vi "main.vi"() -> ()   [LabVIEW 2022 SP3]
uses:
  drawPlate.lvlib
  subvis.lvlib
panel:
  out "x > 0?":bool
  out "depth_max":i32
  out "PowerOff":bool
  in  "GameOver":bool caption="OK"
  out "returnValue":dbl
  out "MoveY":i32
  out "MoveX":i32
  out "nMoves":i32
  in  "pressedJ":i32=21414112
  in  "pressedI":i32=21414112
  out "result":i32
  in  "currentState.pos":i32[][](array[numeric])
  in  "currentState.exist":i32[][](array[numeric])
  in  "availables":i32[][](array[numeric])
  in  "Turn":i32
  in  "mode/difficulty":i32
  out "Tab Control":enum32{"menu", "board"}(tab)
  in  "OL(continue)":bool
  in  "OL(client,white)":bool
  in  "EVE":bool
  in  "OL(host,black)":bool
  in  "PVE":bool
  in  "PVP":bool
  out "mode":string
  in  "7 1":bool
  in  "7 0":bool
  in  "6 1":bool
  in  "6 0":bool
  in  "5 1":bool
  in  "5 0":bool
  in  "4 1":bool
  in  "4 0":bool
  in  "3 1":bool
  in  "3 0":bool
  in  "2 1":bool
  in  "2 0":bool
  in  "1 1":bool
  in  "1 0":bool
  in  "0 1":bool
  in  "7 7":bool
  in  "7 6":bool
  in  "7 5":bool
  in  "7 4":bool
  in  "7 3":bool
  in  "7 2":bool
  in  "6 7":bool
  in  "6 6":bool
  in  "6 5":bool
  in  "6 4":bool
  in  "6 3":bool
  in  "6 2":bool
  in  "5 7":bool
  in  "5 6":bool
  in  "5 5":bool
  in  "5 4":bool
  in  "5 3":bool
  in  "5 2":bool
  in  "4 7":bool
  in  "4 6":bool
  in  "4 5":bool
  in  "4 4":bool
  in  "4 3":bool
  in  "4 2":bool
  in  "3 7":bool
  in  "3 6":bool
  in  "3 5":bool
  in  "3 4":bool
  in  "3 3":bool
  in  "3 2":bool
  in  "2 7":bool
  in  "2 6":bool
  in  "2 5":bool
  in  "2 4":bool
  in  "2 3":bool
  in  "2 2":bool
  in  "0 7":bool
  in  "0 6":bool
  in  "0 5":bool
  in  "0 4":bool
  in  "0 3":bool
  in  "0 2":bool
  in  "1 7":bool
  in  "1 6":bool
  in  "1 5":bool
  in  "1 4":bool
  in  "1 3":bool
  in  "1 2":bool
  in  "0 0":bool
  out "board":picture
  out "Who's turn":string
  in  "GiveUp?":bool
  out "getFromNet":bool
  out "putToNet":bool
  # "等待對方中"
  # "資料上傳中"
  # "連線模式:此二任一亮著代\n表正在將資料上傳或是等\n待下載資料，請勿急著下\n下一手，會當掉。"
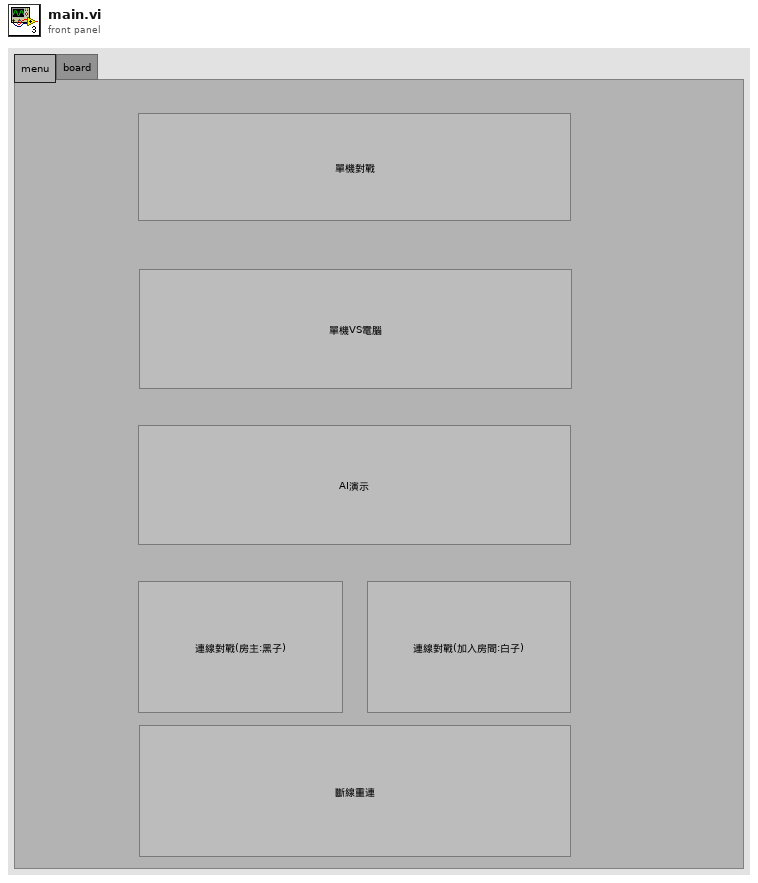
[diagram p1: front panel]
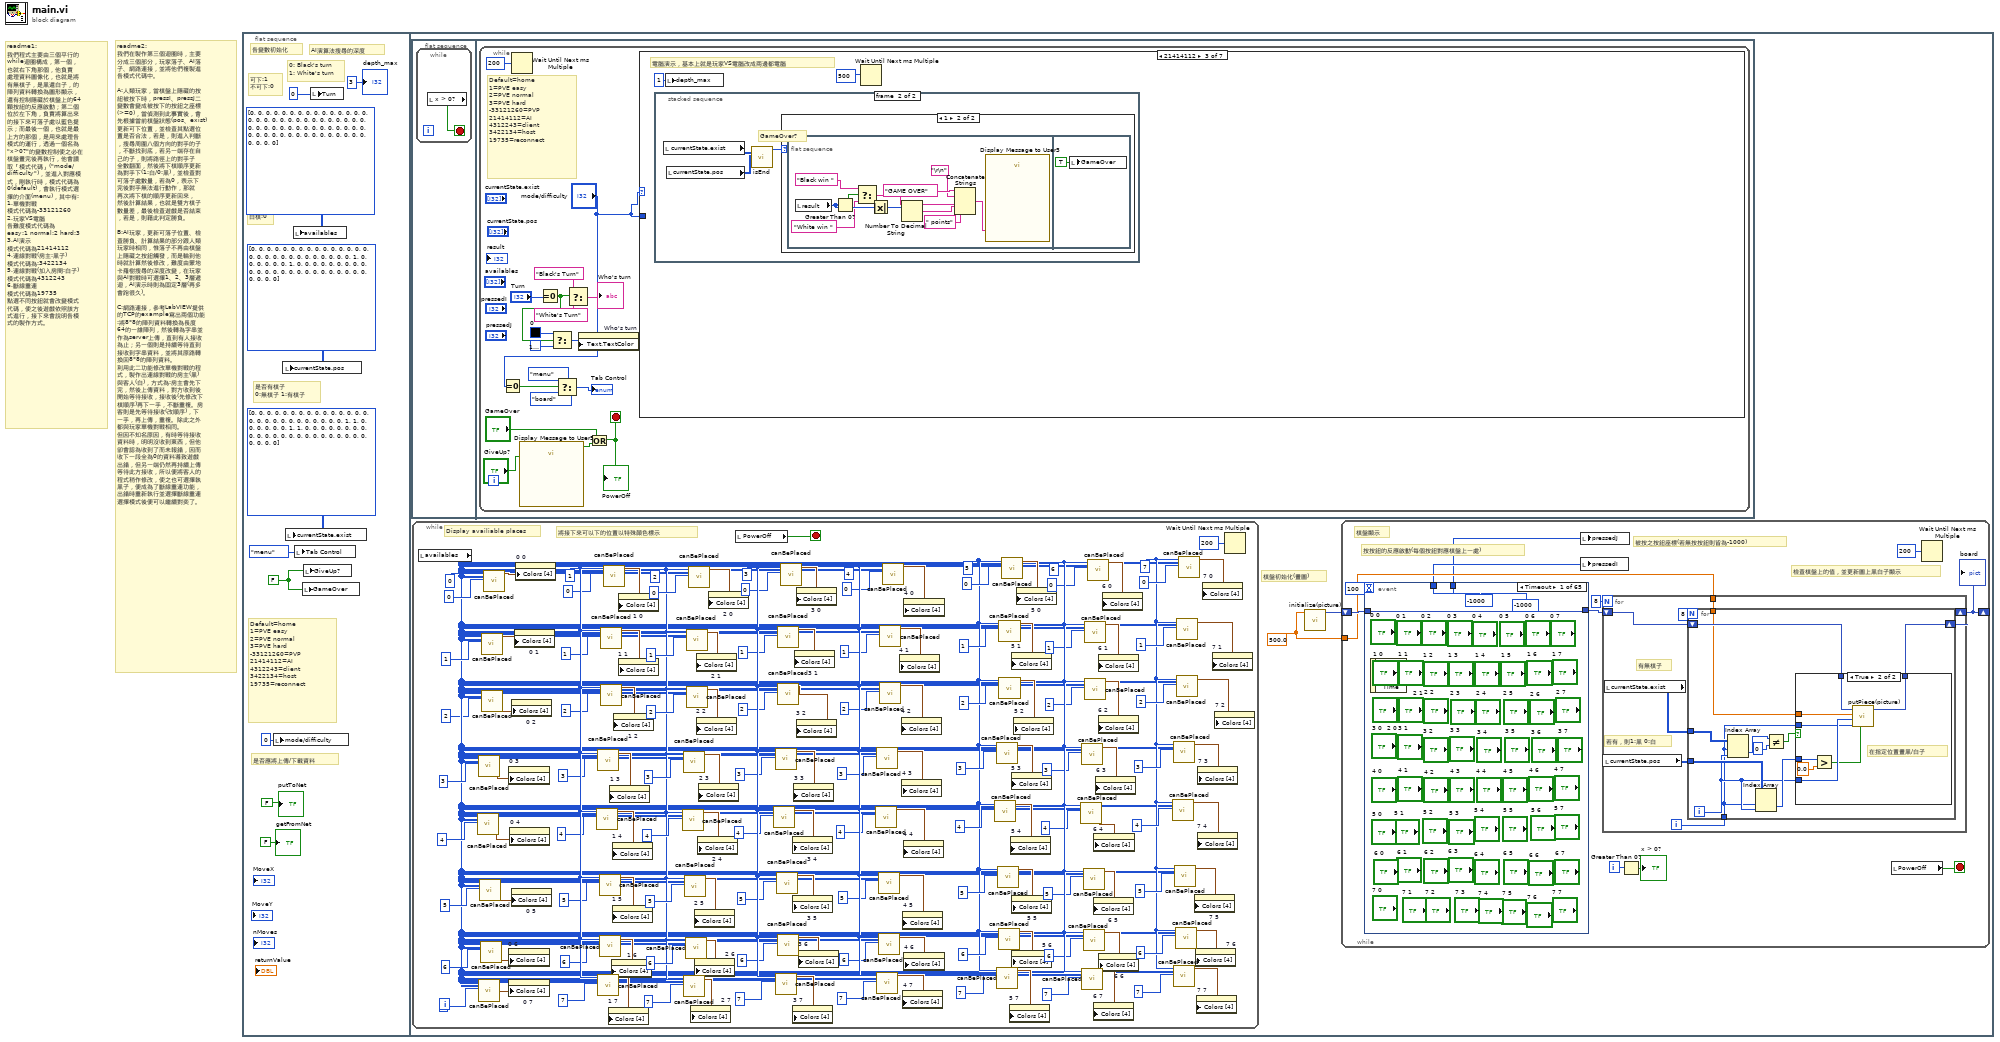
[diagram p0: block diagram]
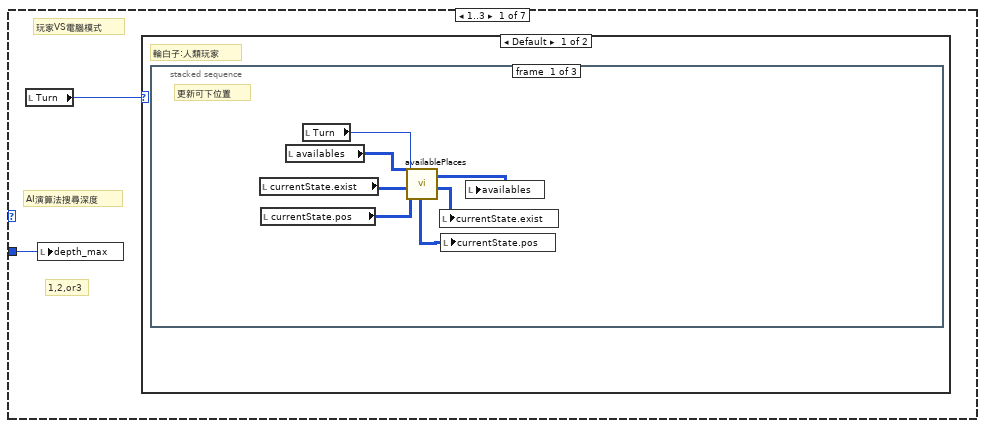
[diagram p2: hidden frame]
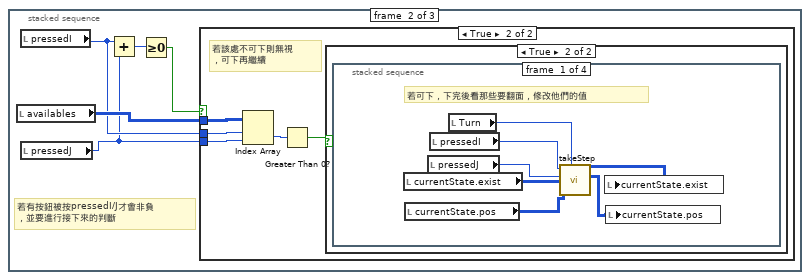
[diagram p3: hidden frame]
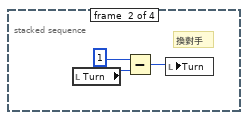
[diagram p6: hidden frame]
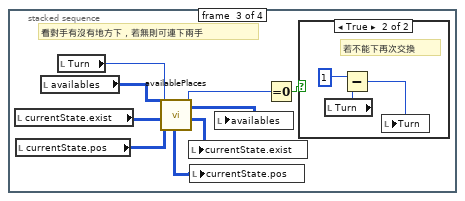
[diagram p7: hidden frame]
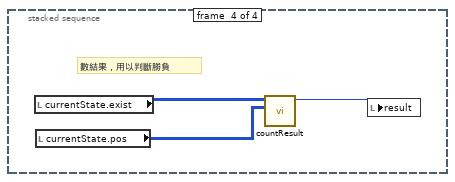
[diagram p9: hidden frame]
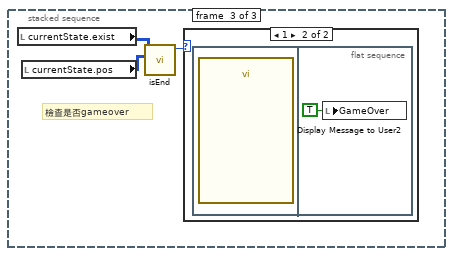
[diagram p10: hidden frame]
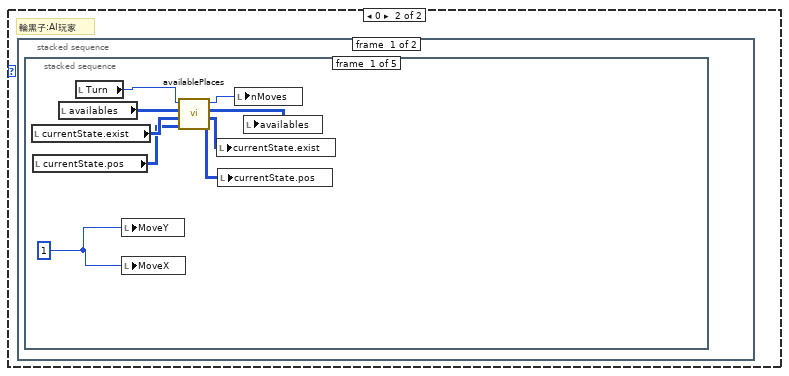
[diagram p12: hidden frame]
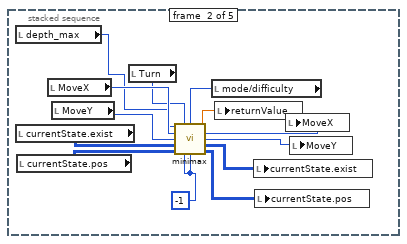
[diagram p13: hidden frame]
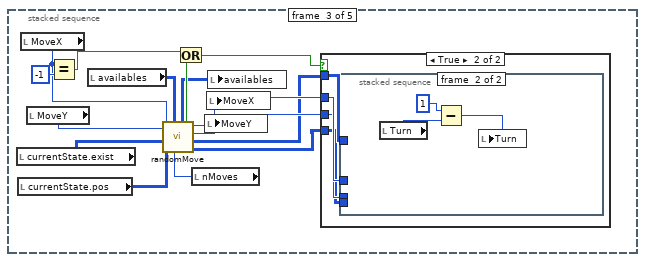
[diagram p14: hidden frame]
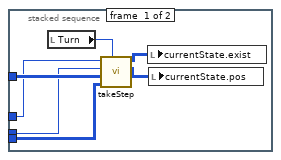
[diagram p16: hidden frame]
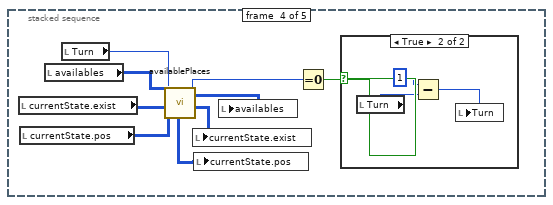
[diagram p17: hidden frame]
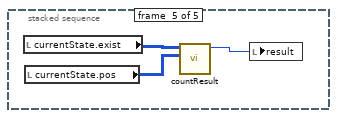
[diagram p19: hidden frame]
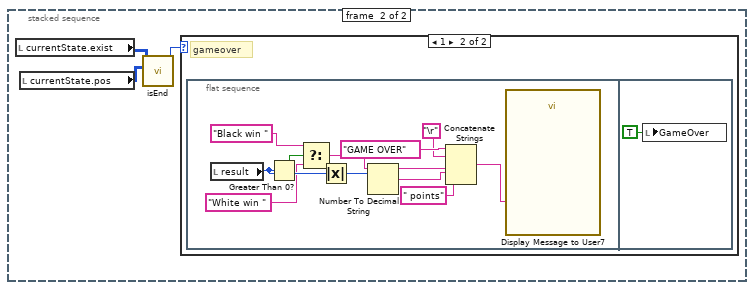
[diagram p20: hidden frame]
diagram:
  # "readme2:\n我們在製作第三個迴圈時，主要\n分成三個部分，玩家落子、AI落\n子、網路連接，並將他們複製進\n各模式代碼中。\n\nA:人類玩家，當棋盤上隱藏的按\n紐被按下時，pressI、pressJ二\n變數會變成被按下的按鈕之座標\n(>=0)，當偵測到此事實後，會\n先根據當前棋盤狀態(pos、exist)\n更新可下位置，並檢查其點選位\n置是否合法，若是，則進入判斷\n，搜尋周圍八個方向的對手的子\n，不斷找到底，若另一端存在自\n己的子，則將路徑上的對手子\n全數翻面，然後將下棋順序更新\n為對手下(1:白/0:黑)，並檢查對\n可落子處數量，若為0，表示下\n完後對手無法進行動作，那就\n再次將下棋的順序更新回來，\n然後計算結果，也就是雙方棋子\n數量差，最後檢查遊戲是否結束\n，若是，則藉此判定勝負。\n\nB:AI玩家，更新可落子位置、檢\n查勝負、計算結果的部分跟人類\n玩家時相同，惟落子不再由棋盤\n上隱藏之按鈕觸發，而是輪到他\n時就計算然後修改，難度由蒙地\n卡羅樹搜尋的深度改變，在玩家\n與AI對戰時可選擇1、2、3層遞\n迴，AI演示時則為固定3層(再多\n會跑很久)。\n\nC:網路連接，參考LabVIEW提供\n的TCP的example寫出兩個功能\n:將8*8的陣列資料轉換為長度\n64的一維陣列，然後轉為字串並\n作為server上傳，直到有人接收\n為止；另一個則是持續等待直到\n接收到字串資料，並將其原路轉\n換回8*8的陣列資料。\n利用此二功能修改單機對戰的程\n式，製作出連線對戰的房主(黑)\n與客人(白)，方式為:房主會先下\n完，然後上傳資料，對方收到後\n開始等待接收，接收後(先修改下\n棋順序)再下一手，不斷重複。房\n客則是先等待接收(改順序)，下\n一手，再上傳，重複。除此之外\n都與玩家單機對戰相同。\n但因不知名原因，有時等待接收\n資料時，明明沒收到東西，但他\n卻會認為收到了而未報錯，因而\n收下一段全為0的資料導致遊戲\n出錯，但另一端仍然再持續上傳\n等待此方接收，所以便將客人的\n程式稍作修改，使之也可選擇執\n黑子，便成為了斷線重連功能，\n出錯時重新執行並選擇斷線重連\n選擇模式後便可以繼續對奕了。"
  # "readme1:\n我們程式主要由三個平行的\nwhile迴圈構成，第一個，\n也就右下角那個，他負責\n處理資料圖像化，也就是將\n有無棋子，是黑還白子，的\n陣列資料轉換為圖形顯示，\n還有控制隱藏於棋盤上的64\n顆按紐的反應啟動；第二個\n位於左下角，負責將算出來\n的接下來可落子處以藍色提\n示；而最後一個，也就是最\n上方的那個，是用來處理各\n模式的運行，透過一個名為\n\"x>0?\"的變數控制使之必在\n棋盤畫完後再執行，他會讀\n取「模式代碼」(\"mode/\ndifficulty\")，並進入對應模\n式，剛執行時，模式代碼為\n0(default)，會執行模式選\n擇的介面(menu)，其中有:\n1.單機對戰\n模式代碼為-33121260\n2.玩家VS電腦\n各難度模式代碼為\neasy:1 normal:2 hard:3\n3.AI演示\n模式代碼為21414112\n4.連線對戰(房主:黑子)\n模式代碼為:3422134\n5.連線對戰(加入房間:白子)\n模式代碼為4312243\n6.斷線重連\n模式代碼為19735\n點選不同按鈕就會改變模式\n代碼，使之後遊戲依照該方\n式進行，接下來會說明各模\n式的製作方式。"
  n1 = flat-sequence {
    frame #0 {
      w7 = FALSE ("powerOff")
      # "是否應將上傳/下載資料"
      # "可下:1\n不可下:0"
      # "Default=home\n1=PVE easy\n2=PVE normal\n3=PVE hard\n-33121260=PVP\n21414112=AI\n4312243=client\n3422134=host\n19735=reconnect"
      # "各變數初始化"
      # "AI演算法搜尋的深度"
      # "0: Black's turn\n1: White's turn"
      # "黑棋:1\n白棋:0"
      # "是否有棋子\n0:無棋子 1:有棋子"
      n2 = local write "mode/difficulty"(0 ("mode/difficulty")) -> ()
      n3 = local write "currentState.pos"(i32[][] [[0, 0, 0, 0, 0, 0, 0, 0], [0, 0, 0, 0, 0, 0, 0, 0], [0, 0, 0, 0, 0, 0, 0, 0], [0, 0, 0, 0, 1, 0, 0, 0], [0, 0, 0, 1, 0, 0, 0, 0], [0, 0, 0, 0, 0, 0, 0, 0], [0, 0, 0, 0, 0, 0, 0, 0], [0, 0, 0, 0, 0, 0, 0, 0]] ("value")) -> ()
      n4 = local write "currentState.exist"(i32[][] [[0, 0, 0, 0, 0, 0, 0, 0], [0, 0, 0, 0, 0, 0, 0, 0], [0, 0, 0, 0, 0, 0, 0, 0], [0, 0, 0, 1, 1, 0, 0, 0], [0, 0, 0, 1, 1, 0, 0, 0], [0, 0, 0, 0, 0, 0, 0, 0], [0, 0, 0, 0, 0, 0, 0, 0], [0, 0, 0, 0, 0, 0, 0, 0]] ("value")) -> ()
      n5 = local write "availables"(i32[][] [[0, 0, 0, 0, 0, 0, 0, 0], [0, 0, 0, 0, 0, 0, 0, 0], [0, 0, 0, 0, 0, 0, 0, 0], [0, 0, 0, 0, 0, 0, 0, 0], [0, 0, 0, 0, 0, 0, 0, 0], [0, 0, 0, 0, 0, 0, 0, 0], [0, 0, 0, 0, 0, 0, 0, 0], [0, 0, 0, 0, 0, 0, 0, 0]] ("value")) -> ()
      n6 = local write "Tab Control"(enum32{"menu", "board"}."menu" ("Tab Control")) -> ()
      n7 = local write "GameOver"(w7) -> ()
      n8 = local write "GiveUp?"(w7) -> ()
      n9 = local write "Turn"(0 ("redTurn")) -> ()
      "depth_max" <- 3 ("depth_max")
      "getFromNet" <- FALSE ("getFromNet")
      "putToNet" <- FALSE ("putToNet")
    }
    frame #1 {
      w11 = 500.0 ("picture size")
      # "棋盤初始化(畫圖)"
      n10 = flat-sequence {
        frame #0 {
          n11 = while {
            stop <- w152 stop-if-true
            n12 = local read "x > 0?"() -> (w152:bool)
          }
        }
        frame #1 {
          n13 = while {
            stop <- w163 stop-if-true
            # "Default=home\n1=PVE easy\n2=PVE normal\n3=PVE hard\n-33121260=PVP\n21414112=AI\n4312243=client\n3422134=host\n19735=reconnect"
            n14 = Equal To 0?(x="mode/difficulty") -> (x = 0?=w168:bool)
            n15 = Wait Until Next ms Multiple(millisecond multiple=u32 200) -> ()  [unwired: 1 out]
            n16 = call "Display Message to User5"("Enable"="GiveUp?") -> ("OK"=w165:bool)  [unwired: 9 in, 1 out]
            n17 = Equal To 0?(x="Turn") -> (x = 0?=w158:bool)
            n18 = Select(t=u32 0 ("Text.Text Colors:Text Color"), s=w158, f=u32 16777225 ("Text.Text Colors:Text Color")) -> (s? t:f=w157:u32)
            n19 = Select(t=enum32{"menu", "board"}."menu" ("Tab Control"), s=w168, f=enum32{"menu", "board"}."board" ("Tab Control")) -> (s? t:f=→"Tab Control":enum32{"menu", "board"})
            n20 = Select(t="Black's Turn", s=w158, f="White's Turn") -> (s? t:f=→"Who's turn":string)
            n21 = property on="Who's turn" class="Str"("Text.TextColor"=w157) -> ()  [unwired: 2 in, 2 out]
            n22 = Or(x="GameOver", y=w165) -> (x .or. y?=w163:bool)
            "PowerOff" <- w163
            n23 = case shown="21414112" "mode/difficulty" {
              tunnel: "mode/difficulty" -> [w171 _ _ _ _ _ _]
              frame 1..3 {
                # "1,2,or3"
                # "AI演算法搜尋深度"
                # "玩家VS電腦模式"
                n24 = local read "Turn"() -> (w172:i32)
                n25 = local write "depth_max"(w171) -> ()
                n26 = case shown="Default" w172 {
                  frame Default {
                    # "輪白子:人類玩家"
                    n27 = stacked-sequence {
                      frame #0 {
                        # "更新可下位置"
                        n28 = local read "currentState.exist"() -> (w174:i32[][])
                        n29 = local read "currentState.pos"() -> (w173:i32[][])
                        n30 = local read "availables"() -> (w175:i32[][])
                        n31 = local read "Turn"() -> (w176:i32)
                        n32 = call "availablePlaces.vi"("pos"=w173, "exist"=w174, "available"=w175, "redTurn"=w176) -> ("posNew"=w179:i32[][], "existNew"=w178:i32[][], "availableNew"=w177:i32[][])  [unwired: 4 in, 1 out]
                        n33 = local write "currentState.exist"(w178) -> ()
                        n34 = local write "currentState.pos"(w179) -> ()
                        n35 = local write "availables"(w177) -> ()
                      }
                      frame #1 {
                        # "若有按鈕被按pressedI/J才會非負\n，並要進行接下來的判斷"
                        n36 = local read "availables"() -> (w183:i32[][])
                        n37 = local read "pressedI"() -> (w181:i32)
                        n38 = local read "pressedJ"() -> (w180:i32)
                        n39 = Add(x=w181, y=w180) -> (x+y=w184:i32)
                        n40 = Greater Or Equal To 0?(x=w184) -> (x >= 0?=w182:bool)
                        n41 = case shown="True" w182 {
                          tunnel: w183 -> [_ w189]
                          tunnel: w181 -> [_ w188]
                          tunnel: w180 -> [_ w187]
                          frame False {
                          }
                          frame True {
                            # "若該處不可下則無視\n，可下再繼續"
                            n42 = Index Array(array=w189, index (row)=w188, index (col)=w187) -> (element=w185:i32)
                            n43 = Greater Than 0?(x=w185) -> (x > 0?=w186:bool)
                            n44 = case shown="True" w186 {
                              frame False {
                              }
                              frame True {
                                n45 = stacked-sequence {
                                frame #0 {
                                # "若可下，下完後看那些要翻面，修改他們的值"
                                n46 = local read "currentState.exist"() -> (w195:i32[][])
                                n47 = local read "currentState.pos"() -> (w194:i32[][])
                                n48 = local read "pressedJ"() -> (w190:i32)
                                n49 = local read "pressedI"() -> (w191:i32)
                                n50 = local read "Turn"() -> (w196:i32)
                                n51 = call "takeStep.vi"("redTurn"=w196, "pos"=w194, "exist"=w195, "j"=w190, "i"=w191) -> ("posNew"=w192:i32[][], "existNew"=w193:i32[][])  [unwired: 4 in, 1 out]
                                n52 = local write "currentState.exist"(w193) -> ()
                                n53 = local write "currentState.pos"(w192) -> ()
                                }
                                frame #1 {
                                # "換對手"
                                n54 = local read "Turn"() -> (w199:i32)
                                n55 = Subtract(x=1 ("y"), y=w199) -> (x-y=w197:i32)
                                n56 = local write "Turn"(w197) -> ()
                                }
                                frame #2 {
                                # "看對手有沒有地方下，若無則可連下兩手"
                                n57 = local read "currentState.exist"() -> (w202:i32[][])
                                n58 = local read "currentState.pos"() -> (w201:i32[][])
                                n59 = local read "availables"() -> (w203:i32[][])
                                n60 = local read "Turn"() -> (w204:i32)
                                n61 = call "availablePlaces.vi"("pos"=w201, "exist"=w202, "available"=w203, "redTurn"=w204) -> ("posNew"=w207:i32[][], "existNew"=w206:i32[][], "availableNew"=w205:i32[][], "count"=w208:i32)  [unwired: 4 in]
                                n62 = local write "currentState.exist"(w206) -> ()
                                n63 = local write "currentState.pos"(w207) -> ()
                                n64 = local write "availables"(w205) -> ()
                                n65 = Equal To 0?(x=w208) -> (x = 0?=w200:bool)
                                n66 = case shown="True" w200 {
                                frame False {
                                }
                                frame True {
                                # "若不能下再次交換"
                                n67 = local read "Turn"() -> (w210:i32)
                                n68 = Subtract(x=1 ("y"), y=w210) -> (x-y=w209:i32)
                                n69 = local write "Turn"(w209) -> ()
                                }
                                }
                                }
                                frame #3 {
                                # "數結果，用以判斷勝負"
                                n70 = local read "currentState.exist"() -> (w213:i32[][])
                                n71 = local read "currentState.pos"() -> (w214:i32[][])
                                n72 = call "countResult.vi"("pos"=w214, "exist"=w213) -> ("result"=w212:i32)  [unwired: 9 in]
                                n73 = local write "result"(w212) -> ()
                                }
                                }
                              }
                            }
                          }
                        }
                      }
                      frame #2 {
                        # "檢查是否gameover"
                        n74 = local read "currentState.exist"() -> (w217:i32[][])
                        n75 = local read "currentState.pos"() -> (w216:i32[][])
                        n76 = call "isEnd.vi"("pos"=w216, "exist"=w217) -> ("isEnd"=w215:i16)  [unwired: 9 in]
                        n77 = case shown="1" w215 {
                          frame 0, Default {
                          }
                          frame 1 {
                            n78 = flat-sequence {
                              frame #0 {
                                n79 = call "Display Message to User2"() -> ()  [unwired: 10 in, 2 out]
                              }
                              frame #1 {
                                n80 = local write "GameOver"(TRUE ("PowerOff")) -> ()
                              }
                            }
                          }
                        }
                      }
                    }
                  }
                  frame 0 {
                    # "輪黑子:AI玩家"
                    n81 = stacked-sequence {
                      frame #0 {
                        n82 = stacked-sequence {
                          frame #0 {
                            w220 = 1
                            n83 = local read "currentState.exist"() -> (w227:i32[][])
                            n84 = local read "currentState.pos"() -> (w226:i32[][])
                            n85 = local read "availables"() -> (w224:i32[][])
                            n86 = local read "Turn"() -> (w225:i32)
                            n87 = local write "MoveY"(w220) -> ()
                            n88 = local write "MoveX"(w220) -> ()
                            n89 = call "availablePlaces.vi"("pos"=w226, "exist"=w227, "available"=w224, "redTurn"=w225) -> ("posNew"=w221:i32[][], "existNew"=w222:i32[][], "availableNew"=w223:i32[][], "count"=w219:i32)  [unwired: 4 in]
                            n90 = local write "currentState.exist"(w222) -> ()
                            n91 = local write "currentState.pos"(w221) -> ()
                            n92 = local write "nMoves"(w219) -> ()
                            n93 = local write "availables"(w223) -> ()
                          }
                          frame #1 {
                            w229 = -1 ("alpha")
                            n94 = local read "depth_max"() -> (w228:i32)
                            n95 = local read "currentState.exist"() -> (w240:i32[][])
                            n96 = local read "currentState.pos"() -> (w239:i32[][])
                            n97 = local read "MoveX"() -> (w237:i32)
                            n98 = local read "MoveY"() -> (w238:i32)
                            n99 = local read "Turn"() -> (w236:i32)
                            n100 = local read "mode/difficulty"() -> (w235:i32)
                            n101 = call "minimax.vi"("depth"=w228, "redTurn"=w236, "mode/difficulty"=w235, "mX"=w237, "mY"=w238, "exist"=w240, "pos"=w239, "alpha"=w229, "beta"=w229) -> ("minimax"=w230:dbl, "mXnew"=w231:i32, "mYnew"=w232:i32, "existNew"=w233:i32[][], "posNew"=w234:i32[][])  [unwired: 2 in]
                            n102 = local write "returnValue"(w230) -> ()
                            n103 = local write "currentState.exist"(w233) -> ()
                            n104 = local write "currentState.pos"(w234) -> ()
                            n105 = local write "MoveX"(w231) -> ()
                            n106 = local write "MoveY"(w232) -> ()
                          }
                          frame #2 {
                            n107 = local read "currentState.exist"() -> (w252:i32[][])
                            n108 = local read "currentState.pos"() -> (w251:i32[][])
                            n109 = local read "MoveX"() -> (w253:i32)
                            n110 = local read "MoveY"() -> (w254:i32)
                            n111 = Equal?(x=w253, y=-1) -> (x = y?=w247:bool)
                            n112 = local read "availables"() -> (w250:i32[][])
                            n113 = local read "nMoves"() -> (w245:i32)
                            n114 = call "randomMove.vi"("nMoves"=w245, "availables"=w250, "pos"=w251, "exist"=w252, "mY"=w254, "mX"=w253) -> ("posNew"=w241:i32[][], "existNew"=w242:i32[][], "mYNew"=w243:i32, "mXNew"=w244:i32, "randomMove"=w248:bool, "availablesNew"=w246:i32[][])
                            n115 = Or(x=w247, y=w248) -> (x .or. y?=w249:bool)
                            n116 = local write "MoveY"(w243) -> ()
                            n117 = local write "MoveX"(w244) -> ()
                            n118 = local write "availables"(w246) -> ()
                            n119 = case shown="True" w249 {
                              tunnel: w242 -> [_ w259]
                              tunnel: w241 -> [_ w256]
                              tunnel: w244 -> [_ w258]
                              tunnel: w243 -> [_ w257]
                              frame False {
                              }
                              frame True {
                                n120 = stacked-sequence {
                                tunnel: w259 -> [w266 _]
                                tunnel: w258 -> [w264 _]
                                tunnel: w257 -> [w263 _]
                                tunnel: w256 -> [w260 _]
                                frame #0 {
                                n121 = local read "Turn"() -> (w265:i32)
                                n122 = call "takeStep.vi"("redTurn"=w265, "pos"=w260, "exist"=w266, "j"=w263, "i"=w264) -> ("posNew"=w261:i32[][], "existNew"=w262:i32[][])  [unwired: 4 in, 1 out]
                                n123 = local write "currentState.exist"(w262) -> ()
                                n124 = local write "currentState.pos"(w261) -> ()
                                }
                                frame #1 {
                                n125 = local read "Turn"() -> (w268:i32)
                                n126 = Subtract(x=1, y=w268) -> (x-y=w267:i32)
                                n127 = local write "Turn"(w267) -> ()
                                }
                                }
                              }
                            }
                          }
                          frame #3 {
                            n128 = local read "currentState.exist"() -> (w277:i32[][])
                            n129 = local read "currentState.pos"() -> (w278:i32[][])
                            n130 = local read "availables"() -> (w276:i32[][])
                            n131 = local read "Turn"() -> (w275:i32)
                            n132 = call "availablePlaces.vi"("pos"=w278, "exist"=w277, "available"=w276, "redTurn"=w275) -> ("posNew"=w272:i32[][], "existNew"=w273:i32[][], "availableNew"=w274:i32[][], "count"=w271:i32)  [unwired: 4 in]
                            n133 = local write "currentState.exist"(w273) -> ()
                            n134 = local write "currentState.pos"(w272) -> ()
                            n135 = local write "availables"(w274) -> ()
                            n136 = Equal To 0?(x=w271) -> (x = 0?=w270:bool)
                            n137 = case shown="True" w270 {
                              frame False {
                              }
                              frame True {
                                n138 = local read "Turn"() -> (w281:i32)
                                n139 = Subtract(x=1, y=w281) -> (x-y=w280:i32)
                                n140 = local write "Turn"(w280) -> ()
                              }
                            }
                          }
                          frame #4 {
                            n141 = local read "currentState.exist"() -> (w284:i32[][])
                            n142 = local read "currentState.pos"() -> (w283:i32[][])
                            n143 = call "countResult.vi"("pos"=w283, "exist"=w284) -> ("result"=w282:i32)  [unwired: 9 in]
                            n144 = local write "result"(w282) -> ()
                          }
                        }
                      }
                      frame #1 {
                        n145 = local read "currentState.exist"() -> (w287:i32[][])
                        n146 = local read "currentState.pos"() -> (w286:i32[][])
                        n147 = call "isEnd.vi"("pos"=w286, "exist"=w287) -> ("isEnd"=w285:i16)  [unwired: 9 in]
                        n148 = case shown="1" w285 {
                          frame 0, Default {
                          }
                          frame 1 {
                            # "gameover"
                            n149 = flat-sequence {
                              frame #0 {
                                n150 = local read "result"() -> (w296:i32)
                                n151 = Greater Than 0?(x=w296) -> (x > 0?=w294:bool)
                                n152 = Select(t="Black win ", s=w294, f="White win ") -> (s? t:f=w295:string)
                                n153 = Absolute Value(x=w296) -> (abs(x)=w297:i32)
                                n154 = Number To Decimal String(number=w297) -> (decimal integer string=w298:string)  [unwired: 1 in]
                                n155 = Concatenate Strings("GAME OVER", "\r", w295, w298, " points" ("string")) -> (w290:string)
                                n156 = call "Display Message to User7"("Message"=w290) -> ()  [unwired: 9 in, 2 out]
                              }
                              frame #1 {
                                n157 = local write "GameOver"(TRUE ("PowerOff")) -> ()
                              }
                            }
                          }
                        }
                      }
                    }
                  }
                }
              }
              frame -33121260 {
                # "PVP，基本上就是玩家VS電腦的東西改成只有玩家"
                n158 = stacked-sequence {
                  frame #0 {
                    n159 = stacked-sequence {
                      frame #0 {
                        # "更新可下位置"
                        n160 = local read "currentState.exist"() -> (w301:i32[][])
                        n161 = local read "currentState.pos"() -> (w300:i32[][])
                        n162 = local read "availables"() -> (w302:i32[][])
                        n163 = local read "Turn"() -> (w303:i32)
                        n164 = call "availablePlaces.vi"("pos"=w300, "exist"=w301, "available"=w302, "redTurn"=w303) -> ("posNew"=w306:i32[][], "existNew"=w305:i32[][], "availableNew"=w304:i32[][])  [unwired: 4 in, 1 out]
                        n165 = local write "currentState.exist"(w305) -> ()
                        n166 = local write "currentState.pos"(w306) -> ()
                        n167 = local write "availables"(w304) -> ()
                      }
                      frame #1 {
                        n168 = local read "pressedI"() -> (w308:i32)
                        n169 = local read "pressedJ"() -> (w307:i32)
                        n170 = local read "availables"() -> (w310:i32[][])
                        n171 = Add(x=w308, y=w307) -> (x+y=w311:i32)
                        n172 = Greater Or Equal To 0?(x=w311) -> (x >= 0?=w309:bool)
                        n173 = case shown="True" w309 {
                          tunnel: w310 -> [_ w316]
                          tunnel: w308 -> [_ w315]
                          tunnel: w307 -> [_ w314]
                          frame False {
                          }
                          frame True {
                            # "是否合法"
                            n174 = Index Array(array=w316, index (row)=w315, index (col)=w314) -> (element=w312:i32)
                            n175 = Greater Than 0?(x=w312) -> (x > 0?=w313:bool)
                            n176 = case shown="True" w313 {
                              frame False {
                              }
                              frame True {
                                n177 = stacked-sequence {
                                frame #0 {
                                n178 = local read "currentState.exist"() -> (w322:i32[][])
                                n179 = local read "currentState.pos"() -> (w321:i32[][])
                                n180 = local read "pressedJ"() -> (w317:i32)
                                n181 = local read "pressedI"() -> (w318:i32)
                                n182 = local read "Turn"() -> (w323:i32)
                                n183 = call "takeStep.vi"("redTurn"=w323, "pos"=w321, "exist"=w322, "j"=w317, "i"=w318) -> ("posNew"=w319:i32[][], "existNew"=w320:i32[][])  [unwired: 4 in, 1 out]
                                n184 = local write "currentState.exist"(w320) -> ()
                                n185 = local write "currentState.pos"(w319) -> ()
                                }
                                frame #1 {
                                n186 = local read "Turn"() -> (w326:i32)
                                n187 = Subtract(x=1 ("y"), y=w326) -> (x-y=w324:i32)
                                n188 = local write "Turn"(w324) -> ()
                                }
                                frame #2 {
                                n189 = local read "currentState.exist"() -> (w329:i32[][])
                                n190 = local read "currentState.pos"() -> (w328:i32[][])
                                n191 = local read "availables"() -> (w330:i32[][])
                                n192 = local read "Turn"() -> (w331:i32)
                                n193 = call "availablePlaces.vi"("pos"=w328, "exist"=w329, "available"=w330, "redTurn"=w331) -> ("posNew"=w334:i32[][], "existNew"=w333:i32[][], "availableNew"=w332:i32[][], "count"=w335:i32)  [unwired: 4 in]
                                n194 = local write "currentState.exist"(w333) -> ()
                                n195 = local write "currentState.pos"(w334) -> ()
                                n196 = local write "availables"(w332) -> ()
                                n197 = Equal To 0?(x=w335) -> (x = 0?=w327:bool)
                                n198 = case shown="True" w327 {
                                frame False {
                                }
                                frame True {
                                n199 = local read "Turn"() -> (w337:i32)
                                n200 = Subtract(x=1 ("y"), y=w337) -> (x-y=w336:i32)
                                n201 = local write "Turn"(w336) -> ()
                                }
                                }
                                }
                                frame #3 {
                                n202 = local read "currentState.exist"() -> (w340:i32[][])
                                n203 = local read "currentState.pos"() -> (w341:i32[][])
                                n204 = call "countResult.vi"("pos"=w341, "exist"=w340) -> ("result"=w339:i32)  [unwired: 9 in]
                                n205 = local write "result"(w339) -> ()
                                }
                                }
                              }
                            }
                          }
                        }
                      }
                    }
                  }
                  frame #1 {
                    n206 = local read "currentState.exist"() -> (w344:i32[][])
                    n207 = local read "currentState.pos"() -> (w343:i32[][])
                    n208 = call "isEnd.vi"("pos"=w343, "exist"=w344) -> ("isEnd"=w342:i16)  [unwired: 9 in]
                    n209 = case shown="1" w342 {
                      frame 0, Default {
                      }
                      frame 1 {
                        # "gameover"
                        n210 = flat-sequence {
                          frame #0 {
                            n211 = local read "result"() -> (w353:i32)
                            n212 = Greater Than 0?(x=w353) -> (x > 0?=w351:bool)
                            n213 = Select(t="Black win ", s=w351, f="White win ") -> (s? t:f=w352:string)
                            n214 = Absolute Value(x=w353) -> (abs(x)=w354:i32)
                            n215 = Number To Decimal String(number=w354) -> (decimal integer string=w355:string)  [unwired: 1 in]
                            n216 = Concatenate Strings("GAME OVER", "\r\n", w352, w355, " points" ("string")) -> (w347:string)
                            n217 = call "Display Message to User4"("Message"=w347) -> ()  [unwired: 9 in, 2 out]
                          }
                          frame #1 {
                            n218 = local write "GameOver"(TRUE ("PowerOff")) -> ()
                          }
                        }
                      }
                    }
                  }
                }
              }
              frame 21414112 {
                # "電腦演示，基本上就是玩家VS電腦改成兩邊都電腦"
                n219 = stacked-sequence {
                  frame #0 {
                    n220 = stacked-sequence {
                      frame #0 {
                        w360 = 1
                        n221 = local read "currentState.exist"() -> (w367:i32[][])
                        n222 = local read "currentState.pos"() -> (w366:i32[][])
                        n223 = local read "availables"() -> (w364:i32[][])
                        n224 = local read "Turn"() -> (w365:i32)
                        n225 = call "availablePlaces.vi"("pos"=w366, "exist"=w367, "available"=w364, "redTurn"=w365) -> ("posNew"=w361:i32[][], "existNew"=w362:i32[][], "availableNew"=w363:i32[][], "count"=w359:i32)  [unwired: 4 in]
                        n226 = local write "currentState.exist"(w362) -> ()
                        n227 = local write "currentState.pos"(w361) -> ()
                        n228 = local write "nMoves"(w359) -> ()
                        n229 = local write "availables"(w363) -> ()
                        n230 = local write "MoveY"(w360) -> ()
                        n231 = local write "MoveX"(w360) -> ()
                      }
                      frame #1 {
                        w369 = -1 ("alpha")
                        n232 = local read "depth_max"() -> (w368:i32)
                        n233 = local read "currentState.exist"() -> (w380:i32[][])
                        n234 = local read "currentState.pos"() -> (w379:i32[][])
                        n235 = local read "MoveX"() -> (w377:i32)
                        n236 = local read "MoveY"() -> (w378:i32)
                        n237 = local read "Turn"() -> (w376:i32)
                        n238 = local read "mode/difficulty"() -> (w375:i32)
                        n239 = call "minimax.vi"("depth"=w368, "redTurn"=w376, "mode/difficulty"=w375, "mX"=w377, "mY"=w378, "exist"=w380, "pos"=w379, "alpha"=w369, "beta"=w369) -> ("minimax"=w370:dbl, "mXnew"=w371:i32, "mYnew"=w372:i32, "existNew"=w373:i32[][], "posNew"=w374:i32[][])  [unwired: 2 in]
                        n240 = local write "returnValue"(w370) -> ()
                        n241 = local write "currentState.exist"(w373) -> ()
                        n242 = local write "currentState.pos"(w374) -> ()
                        n243 = local write "MoveX"(w371) -> ()
                        n244 = local write "MoveY"(w372) -> ()
                      }
                      frame #2 {
                        n245 = local read "currentState.exist"() -> (w392:i32[][])
                        n246 = local read "currentState.pos"() -> (w391:i32[][])
                        n247 = local read "MoveX"() -> (w393:i32)
                        n248 = local read "MoveY"() -> (w394:i32)
                        n249 = Equal?(x=w393, y=-1) -> (x = y?=w387:bool)
                        n250 = local read "availables"() -> (w390:i32[][])
                        n251 = local read "nMoves"() -> (w385:i32)
                        n252 = call "randomMove.vi"("nMoves"=w385, "availables"=w390, "pos"=w391, "exist"=w392, "mY"=w394, "mX"=w393) -> ("posNew"=w381:i32[][], "existNew"=w382:i32[][], "mYNew"=w383:i32, "mXNew"=w384:i32, "randomMove"=w388:bool, "availablesNew"=w386:i32[][])
                        n253 = Or(x=w387, y=w388) -> (x .or. y?=w389:bool)
                        n254 = local write "MoveY"(w383) -> ()
                        n255 = local write "MoveX"(w384) -> ()
                        n256 = local write "availables"(w386) -> ()
                        n257 = case shown="True" w389 {
                          tunnel: w382 -> [_ w399]
                          tunnel: w381 -> [_ w396]
                          tunnel: w384 -> [_ w398]
                          tunnel: w383 -> [_ w397]
                          frame False {
                          }
                          frame True {
                            n258 = stacked-sequence {
                              tunnel: w399 -> [w406 _]
                              tunnel: w398 -> [w404 _]
                              tunnel: w397 -> [w403 _]
                              tunnel: w396 -> [w400 _]
                              frame #0 {
                                n259 = local read "Turn"() -> (w405:i32)
                                n260 = call "takeStep.vi"("redTurn"=w405, "pos"=w400, "exist"=w406, "j"=w403, "i"=w404) -> ("posNew"=w401:i32[][], "existNew"=w402:i32[][])  [unwired: 4 in, 1 out]
                                n261 = local write "currentState.exist"(w402) -> ()
                                n262 = local write "currentState.pos"(w401) -> ()
                              }
                              frame #1 {
                                n263 = local read "Turn"() -> (w408:i32)
                                n264 = Subtract(x=1, y=w408) -> (x-y=w407:i32)
                                n265 = local write "Turn"(w407) -> ()
                              }
                            }
                          }
                        }
                      }
                      frame #3 {
                        n266 = local read "currentState.exist"() -> (w417:i32[][])
                        n267 = local read "currentState.pos"() -> (w418:i32[][])
                        n268 = local read "availables"() -> (w416:i32[][])
                        n269 = local read "Turn"() -> (w415:i32)
                        n270 = call "availablePlaces.vi"("pos"=w418, "exist"=w417, "available"=w416, "redTurn"=w415) -> ("posNew"=w412:i32[][], "existNew"=w413:i32[][], "availableNew"=w414:i32[][], "count"=w411:i32)  [unwired: 4 in]
                        n271 = local write "currentState.exist"(w413) -> ()
                        n272 = local write "currentState.pos"(w412) -> ()
                        n273 = local write "availables"(w414) -> ()
                        n274 = Equal To 0?(x=w411) -> (x = 0?=w410:bool)
                        n275 = case shown="True" w410 {
                          frame False {
                          }
                          frame True {
                            n276 = local read "Turn"() -> (w421:i32)
                            n277 = Subtract(x=1, y=w421) -> (x-y=w420:i32)
                            n278 = local write "Turn"(w420) -> ()
                          }
                        }
                      }
                      frame #4 {
                        n279 = local read "currentState.exist"() -> (w424:i32[][])
                        n280 = local read "currentState.pos"() -> (w423:i32[][])
                        n281 = call "countResult.vi"("pos"=w423, "exist"=w424) -> ("result"=w422:i32)  [unwired: 9 in]
                        n282 = local write "result"(w422) -> ()
                      }
                    }
                  }
                  frame #1 {
                    # "GameOver?"
                    n283 = local read "currentState.exist"() -> (w427:i32[][])
                    n284 = local read "currentState.pos"() -> (w426:i32[][])
                    n285 = call "isEnd.vi"("pos"=w426, "exist"=w427) -> ("isEnd"=w425:i16)  [unwired: 9 in]
                    n286 = case shown="1" w425 {
                      frame 0, Default {
                      }
                      frame 1 {
                        n287 = flat-sequence {
                          frame #0 {
                            n288 = local read "result"() -> (w436:i32)
                            n289 = Greater Than 0?(x=w436) -> (x > 0?=w434:bool)
                            n290 = Select(t="Black win ", s=w434, f="White win ") -> (s? t:f=w435:string)
                            n291 = Absolute Value(x=w436) -> (abs(x)=w437:i32)
                            n292 = Number To Decimal String(number=w437) -> (decimal integer string=w438:string)  [unwired: 1 in]
                            n293 = Concatenate Strings("GAME OVER", "\r\n", w435, w438, " points" ("string")) -> (w430:string)
                            n294 = call "Display Message to User3"("Message"=w430) -> ()  [unwired: 9 in, 2 out]
                          }
                          frame #1 {
                            n295 = local write "GameOver"(TRUE ("PowerOff")) -> ()
                          }
                        }
                      }
                    }
                  }
                }
                n296 = local write "depth_max"(1 ("depth_max")) -> ()
                n297 = Wait Until Next ms Multiple(millisecond multiple=u32 500) -> ()  [unwired: 1 out]
              }
              frame 4312243 {
                # "網路連線:client，固定執白子，先從網路上接收server的資料，下一子後，自己當作server傳輸資料直到另一端接收，並再次等待從server接收到資料，反覆，其餘同PVP"
                n298 = stacked-sequence {
                  frame #0 {
                    n299 = stacked-sequence {
                      frame #0 {
                        n300 = flat-sequence {
                          frame #0 {
                            # "初始化時令為T"
                            n301 = local read "getFromNet"() -> (w440:bool)
                            n302 = case shown="True" w440 {
                              frame False {
                              }
                              frame True {
                                n303 = flat-sequence {
                                frame #0 {
                                # "傳送/接收的資料類型為currentState的pos+exist，也就是說，2:黑子，1:白子，0:空格，並將其轉換回pos、exist的格式"
                                n304 = call "client.vi"() -> ("value"=w441:i32[][])  [unwired: 10 in, 1 out]
                                n305 = for {
                                tunnel: w441 -> [w445] mode=indexing
                                tunnel: [w443] -> w442 mode=indexing
                                i -> [w444]
                                n306 = for {
                                tunnel: w445 -> [w447] mode=indexing
                                tunnel: w444 -> [w449]
                                tunnel: [w446] -> w443 mode=indexing
                                i -> [w448]
                                n307 = Greater?(x=w447, y=0) -> (0:w450:bool)
                                n308 = case shown="True" w450 {
                                tunnel: w449 -> [_ w457]
                                tunnel: w448 -> [_ w456]
                                tunnel: [w452 w453] -> w446
                                tunnel: w447 -> [w452 w454]
                                frame False {
                                }
                                frame True {
                                n309 = local read "currentState.exist"() -> (w458:i32[][])
                                n310 = Replace Array Subset(array=w458, new element=1 ("new element/subarray"), index (row)=w457, index (col)=w456) -> (w459:i32[][])
                                n311 = Decrement(x=w454) -> (x-1=w453:i32)
                                n312 = local write "currentState.exist"(w459) -> ()
                                }
                                }
                                }
                                }
                                n313 = local write "currentState.pos"(w442) -> ()
                                }
                                frame #1 {
                                n314 = local write "getFromNet"(FALSE ("getFromNet")) -> ()
                                n315 = local write "Turn"(1 ("redTurn")) -> ()
                                }
                                }
                              }
                            }
                          }
                          frame #1 {
                            n316 = local read "currentState.exist"() -> (w464:i32[][])
                            n317 = local read "currentState.pos"() -> (w463:i32[][])
                            n318 = local read "availables"() -> (w465:i32[][])
                            n319 = call "availablePlaces.vi"("pos"=w463, "exist"=w464, "available"=w465, "redTurn"=1) -> ("availableNew"=w466:i32[][])  [unwired: 4 in, 3 out]
                            n320 = local write "availables"(w466) -> ()
                          }
                        }
                      }
                      frame #1 {
                        # "下載資料後更新可下的位置"
                        n321 = local read "currentState.exist"() -> (w468:i32[][])
                        n322 = local read "currentState.pos"() -> (w467:i32[][])
                        n323 = local read "availables"() -> (w469:i32[][])
                        n324 = local read "Turn"() -> (w470:i32)
                        n325 = call "availablePlaces.vi"("pos"=w467, "exist"=w468, "available"=w469, "redTurn"=w470) -> ("availableNew"=w471:i32[][])  [unwired: 4 in, 3 out]
                        n326 = local write "availables"(w471) -> ()
                      }
                      frame #2 {
                        # "等待下棋，下完棋後要將資料送至網路上"
                        n327 = local read "pressedI"() -> (w473:i32)
                        n328 = local read "pressedJ"() -> (w472:i32)
                        n329 = local read "availables"() -> (w475:i32[][])
                        n330 = Add(x=w473, y=w472) -> (x+y=w476:i32)
                        n331 = Greater Or Equal To 0?(x=w476) -> (x >= 0?=w474:bool)
                        n332 = case shown="True" w474 {
                          tunnel: w475 -> [_ w481]
                          tunnel: w473 -> [_ w480]
                          tunnel: w472 -> [_ w479]
                          frame False {
                          }
                          frame True {
                            n333 = Index Array(array=w481, index (row)=w480, index (col)=w479) -> (element=w477:i32)
                            n334 = Greater Than 0?(x=w477) -> (x > 0?=w478:bool)
                            n335 = case shown="True" w478 {
                              frame False {
                                # "error mess."
                                n336 = call "Display Message to User"() -> ()  [unwired: 10 in, 2 out]
                              }
                              frame True {
                                n337 = stacked-sequence {
                                frame #0 {
                                n338 = local read "currentState.exist"() -> (w487:i32[][])
                                n339 = local read "currentState.pos"() -> (w486:i32[][])
                                n340 = local read "pressedJ"() -> (w482:i32)
                                n341 = local read "pressedI"() -> (w483:i32)
                                n342 = local read "Turn"() -> (w488:i32)
                                n343 = call "takeStep.vi"("redTurn"=w488, "pos"=w486, "exist"=w487, "j"=w482, "i"=w483) -> ("posNew"=w484:i32[][], "existNew"=w485:i32[][])  [unwired: 4 in, 1 out]
                                n344 = local write "currentState.exist"(w485) -> ()
                                n345 = local write "currentState.pos"(w484) -> ()
                                }
                                frame #1 {
                                # "下完棋後要將資料送至網路上"
                                n346 = local write "putToNet"(TRUE ("getFromNet")) -> ()
                                }
                                frame #2 {
                                # "換對手"
                                n347 = local read "Turn"() -> (w492:i32)
                                n348 = Subtract(x=1 ("y"), y=w492) -> (x-y=w490:i32)
                                n349 = local write "Turn"(w490) -> ()
                                }
                                frame #3 {
                                n350 = local read "currentState.exist"() -> (w495:i32[][])
                                n351 = local read "currentState.pos"() -> (w494:i32[][])
                                n352 = local read "availables"() -> (w496:i32[][])
                                n353 = local read "Turn"() -> (w497:i32)
                                n354 = call "availablePlaces.vi"("pos"=w494, "exist"=w495, "available"=w496, "redTurn"=w497) -> ("posNew"=w500:i32[][], "existNew"=w499:i32[][], "availableNew"=w498:i32[][], "count"=w501:i32)  [unwired: 4 in]
                                n355 = local write "currentState.exist"(w499) -> ()
                                n356 = local write "currentState.pos"(w500) -> ()
                                n357 = local write "availables"(w498) -> ()
                                n358 = Equal To 0?(x=w501) -> (x = 0?=w493:bool)
                                n359 = case shown="True" w493 {
                                frame False {
                                }
                                frame True {
                                # "若不能下，再次交換"
                                n360 = local read "Turn"() -> (w503:i32)
                                n361 = Subtract(x=1 ("y"), y=w503) -> (x-y=w502:i32)
                                n362 = local write "Turn"(w502) -> ()
                                }
                                }
                                }
                                frame #4 {
                                # "計算結果"
                                n363 = local read "currentState.exist"() -> (w506:i32[][])
                                n364 = local read "currentState.pos"() -> (w507:i32[][])
                                n365 = call "countResult.vi"("pos"=w507, "exist"=w506) -> ("result"=w505:i32)  [unwired: 9 in]
                                n366 = local write "result"(w505) -> ()
                                }
                                }
                              }
                            }
                          }
                        }
                      }
                    }
                  }
                  frame #1 {
                    n367 = local read "currentState.exist"() -> (w510:i32[][])
                    n368 = local read "currentState.pos"() -> (w509:i32[][])
                    n369 = call "isEnd.vi"("pos"=w509, "exist"=w510) -> ("isEnd"=w508:i16)  [unwired: 9 in]
                    n370 = case shown="1" w508 {
                      frame 0, Default {
                      }
                      frame 1 {
                        # "gameover"
                        n371 = flat-sequence {
                          frame #0 {
                            n372 = local read "result"() -> (w519:i32)
                            n373 = Greater Than 0?(x=w519) -> (x > 0?=w517:bool)
                            n374 = Select(t="Black win ", s=w517, f="White win ") -> (s? t:f=w518:string)
                            n375 = Absolute Value(x=w519) -> (abs(x)=w520:i32)
                            n376 = Number To Decimal String(number=w520) -> (decimal integer string=w521:string)  [unwired: 1 in]
                            n377 = Concatenate Strings("GAME OVER", "\r\n", w518, w521, " points" ("string")) -> (w513:string)
                            n378 = call "Display Message to User8"("Message"=w513) -> ()  [unwired: 9 in, 2 out]
                          }
                          frame #1 {
                            n379 = local write "GameOver"(TRUE ("PowerOff")) -> ()
                          }
                        }
                      }
                    }
                  }
                  frame #2 {
                    # "下完後將資料處理(pos+exist)後上傳，並修改getFromNet，使下一輪會等待從網路上接收資料"
                    n380 = local read "putToNet"() -> (w523:bool)
                    n381 = case shown="True" w523 {
                      frame False {
                      }
                      frame True {
                        n382 = flat-sequence {
                          frame #0 {
                            n383 = local read "currentState.exist"() -> (w526:i32[][])
                            n384 = local read "currentState.pos"() -> (w527:i32[][])
                            n385 = for {
                              tunnel: w526 -> [w530] mode=indexing
                              tunnel: w527 -> [w529] mode=indexing
                              tunnel: [w528] -> w525 mode=indexing
                              n386 = for {
                                tunnel: w530 -> [w533] mode=indexing
                                tunnel: w529 -> [w532] mode=indexing
                                tunnel: [w531] -> w528 mode=indexing
                                n387 = Add(x=w533, y=w532) -> (x+y=w531:i32)
                              }
                            }
                            n388 = local write "getFromNet"(TRUE ("getFromNet")) -> ()
                            n389 = call "server.vi"("array"=w525) -> ()  [unwired: 10 in, 1 out]
                          }
                          frame #1 {
                            n390 = local write "putToNet"(FALSE) -> ()
                          }
                        }
                      }
                    }
                  }
                }
              }
              frame 19735 {
                # "斷線重連，基本上與加入房間一樣，只是所執不一定為白子，也會恢復初始狀態，而是要選擇斷線前所執的，由於不知明原因會使一方接收到全空白資料卻未報錯，另一方因無人收取資料仍在進行傳輸，故先接收對方正在傳輸的資料再繼續遊戲即可"
                n391 = stacked-sequence {
                  frame #0 {
                    n392 = stacked-sequence {
                      frame #0 {
                        n393 = flat-sequence {
                          frame #0 {
                            n394 = local read "getFromNet"() -> (w535:bool)
                            n395 = case shown="True" w535 {
                              frame False {
                              }
                              frame True {
                                n396 = flat-sequence {
                                frame #0 {
                                n397 = call "client.vi"() -> ("value"=w536:i32[][])  [unwired: 10 in, 1 out]
                                n398 = for {
                                tunnel: w536 -> [w540] mode=indexing
                                tunnel: [w538] -> w537 mode=indexing
                                i -> [w539]
                                n399 = for {
                                tunnel: w540 -> [w542] mode=indexing
                                tunnel: w539 -> [w544]
                                tunnel: [w541] -> w538 mode=indexing
                                i -> [w543]
                                n400 = Greater?(x=w542, y=0) -> (0:w545:bool)
                                n401 = case shown="True" w545 {
                                tunnel: w544 -> [_ w552]
                                tunnel: w543 -> [_ w551]
                                tunnel: [w547 w548] -> w541
                                tunnel: w542 -> [w547 w549]
                                frame False {
                                }
                                frame True {
                                n402 = local read "currentState.exist"() -> (w553:i32[][])
                                n403 = Replace Array Subset(array=w553, new element=1 ("new element/subarray"), index (row)=w552, index (col)=w551) -> (w554:i32[][])
                                n404 = Decrement(x=w549) -> (x-1=w548:i32)
                                n405 = local write "currentState.exist"(w554) -> ()
                                }
                                }
                                }
                                }
                                n406 = local write "currentState.pos"(w537) -> ()
                                }
                                frame #1 {
                                n407 = local read "Turn"() -> (w555:i32)
                                n408 = local write "getFromNet"(FALSE ("getFromNet")) -> ()
                                n409 = Subtract(x=1 ("redTurn"), y=w555) -> (x-y=w556:i32)
                                n410 = local write "Turn"(w556) -> ()
                                }
                                }
                              }
                            }
                          }
                          frame #1 {
                            n411 = local read "currentState.exist"() -> (w561:i32[][])
                            n412 = local read "currentState.pos"() -> (w560:i32[][])
                            n413 = local read "availables"() -> (w562:i32[][])
                            n414 = local read "Turn"() -> (w559:i32)
                            n415 = call "availablePlaces.vi"("pos"=w560, "exist"=w561, "available"=w562, "redTurn"=w559) -> ("availableNew"=w563:i32[][])  [unwired: 4 in, 3 out]
                            n416 = local write "availables"(w563) -> ()
                          }
                        }
                      }
                      frame #1 {
                        n417 = local read "currentState.exist"() -> (w565:i32[][])
                        n418 = local read "currentState.pos"() -> (w564:i32[][])
                        n419 = local read "availables"() -> (w566:i32[][])
                        n420 = local read "Turn"() -> (w567:i32)
                        n421 = call "availablePlaces.vi"("pos"=w564, "exist"=w565, "available"=w566, "redTurn"=w567) -> ("availableNew"=w568:i32[][])  [unwired: 4 in, 3 out]
                        n422 = local write "availables"(w568) -> ()
                      }
                      frame #2 {
                        n423 = local read "pressedI"() -> (w570:i32)
                        n424 = local read "pressedJ"() -> (w569:i32)
                        n425 = local read "availables"() -> (w572:i32[][])
                        n426 = Add(x=w570, y=w569) -> (x+y=w573:i32)
                        n427 = Greater Or Equal To 0?(x=w573) -> (x >= 0?=w571:bool)
                        n428 = case shown="True" w571 {
                          tunnel: w572 -> [_ w578]
                          tunnel: w570 -> [_ w577]
                          tunnel: w569 -> [_ w576]
                          frame False {
                          }
                          frame True {
                            n429 = Index Array(array=w578, index (row)=w577, index (col)=w576) -> (element=w574:i32)
                            n430 = Greater Than 0?(x=w574) -> (x > 0?=w575:bool)
                            n431 = case shown="True" w575 {
                              frame False {
                                # "error mess."
                                n432 = call "Display Message to User11"() -> ()  [unwired: 10 in, 2 out]
                              }
                              frame True {
                                n433 = stacked-sequence {
                                frame #0 {
                                n434 = local read "currentState.exist"() -> (w584:i32[][])
                                n435 = local read "currentState.pos"() -> (w583:i32[][])
                                n436 = local read "pressedJ"() -> (w579:i32)
                                n437 = local read "pressedI"() -> (w580:i32)
                                n438 = local read "Turn"() -> (w585:i32)
                                n439 = call "takeStep.vi"("redTurn"=w585, "pos"=w583, "exist"=w584, "j"=w579, "i"=w580) -> ("posNew"=w581:i32[][], "existNew"=w582:i32[][])  [unwired: 4 in, 1 out]
                                n440 = local write "currentState.exist"(w582) -> ()
                                n441 = local write "currentState.pos"(w581) -> ()
                                }
                                frame #1 {
                                n442 = local write "putToNet"(TRUE ("getFromNet")) -> ()
                                }
                                frame #2 {
                                n443 = local read "Turn"() -> (w589:i32)
                                n444 = Subtract(x=1 ("y"), y=w589) -> (x-y=w587:i32)
                                n445 = local write "Turn"(w587) -> ()
                                }
                                frame #3 {
                                # "若不能動再次交換"
                                n446 = local read "currentState.exist"() -> (w592:i32[][])
                                n447 = local read "currentState.pos"() -> (w591:i32[][])
                                n448 = local read "availables"() -> (w593:i32[][])
                                n449 = local read "Turn"() -> (w594:i32)
                                n450 = call "availablePlaces.vi"("pos"=w591, "exist"=w592, "available"=w593, "redTurn"=w594) -> ("posNew"=w597:i32[][], "existNew"=w596:i32[][], "availableNew"=w595:i32[][], "count"=w598:i32)  [unwired: 4 in]
                                n451 = local write "currentState.exist"(w596) -> ()
                                n452 = local write "currentState.pos"(w597) -> ()
                                n453 = local write "availables"(w595) -> ()
                                n454 = Equal To 0?(x=w598) -> (x = 0?=w590:bool)
                                n455 = case shown="True" w590 {
                                frame False {
                                }
                                frame True {
                                n456 = local read "Turn"() -> (w600:i32)
                                n457 = Subtract(x=1 ("y"), y=w600) -> (x-y=w599:i32)
                                n458 = local write "Turn"(w599) -> ()
                                }
                                }
                                }
                                frame #4 {
                                n459 = local read "currentState.exist"() -> (w603:i32[][])
                                n460 = local read "currentState.pos"() -> (w604:i32[][])
                                n461 = call "countResult.vi"("pos"=w604, "exist"=w603) -> ("result"=w602:i32)  [unwired: 9 in]
                                n462 = local write "result"(w602) -> ()
                                }
                                }
                              }
                            }
                          }
                        }
                      }
                    }
                  }
                  frame #1 {
                    n463 = local read "currentState.exist"() -> (w607:i32[][])
                    n464 = local read "currentState.pos"() -> (w606:i32[][])
                    n465 = call "isEnd.vi"("pos"=w606, "exist"=w607) -> ("isEnd"=w605:i16)  [unwired: 9 in]
                    n466 = case shown="1" w605 {
                      frame 0, Default {
                      }
                      frame 1 {
                        # "gameover"
                        n467 = flat-sequence {
                          frame #0 {
                            n468 = local read "result"() -> (w616:i32)
                            n469 = Greater Than 0?(x=w616) -> (x > 0?=w614:bool)
                            n470 = Select(t="Black win ", s=w614, f="White win ") -> (s? t:f=w615:string)
                            n471 = Absolute Value(x=w616) -> (abs(x)=w617:i32)
                            n472 = Number To Decimal String(number=w617) -> (decimal integer string=w618:string)  [unwired: 1 in]
                            n473 = Concatenate Strings("GAME OVER", "\r\n", w615, w618, " points" ("string")) -> (w610:string)
                            n474 = call "Display Message to User12"("Message"=w610) -> ()  [unwired: 9 in, 2 out]
                          }
                          frame #1 {
                            n475 = local write "GameOver"(TRUE ("PowerOff")) -> ()
                          }
                        }
                      }
                    }
                  }
                  frame #2 {
                    w621 = -1000 ("pressedJ")
                    n476 = local read "putToNet"() -> (w620:bool)
                    n477 = local write "pressedJ"(w621) -> ()
                    n478 = local write "pressedI"(w621) -> ()
                    n479 = case shown="True" w620 {
                      frame False {
                      }
                      frame True {
                        n480 = flat-sequence {
                          frame #0 {
                            n481 = local read "currentState.exist"() -> (w624:i32[][])
                            n482 = local read "currentState.pos"() -> (w625:i32[][])
                            n483 = for {
                              tunnel: w624 -> [w628] mode=indexing
                              tunnel: w625 -> [w627] mode=indexing
                              tunnel: [w626] -> w623 mode=indexing
                              n484 = for {
                                tunnel: w628 -> [w631] mode=indexing
                                tunnel: w627 -> [w630] mode=indexing
                                tunnel: [w629] -> w626 mode=indexing
                                n485 = Add(x=w631, y=w630) -> (x+y=w629:i32)
                              }
                            }
                            n486 = local write "getFromNet"(TRUE ("getFromNet")) -> ()
                            n487 = call "server.vi"("array"=w623) -> ()  [unwired: 10 in, 1 out]
                          }
                          frame #1 {
                            n488 = local write "putToNet"(FALSE) -> ()
                          }
                        }
                      }
                    }
                  }
                }
              }
              frame 3422134 {
                # "網路連線:host，固定執黑子，先下完一手後，開始作為server傳輸資料，對方接收後改為作為client接收資料，接到後在下一手，反覆，其餘同玩家VS玩家"
                n489 = stacked-sequence {
                  frame #0 {
                    n490 = stacked-sequence {
                      frame #0 {
                        n491 = local read "currentState.exist"() -> (w634:i32[][])
                        n492 = local read "currentState.pos"() -> (w633:i32[][])
                        n493 = local read "availables"() -> (w635:i32[][])
                        n494 = local read "Turn"() -> (w636:i32)
                        n495 = call "availablePlaces.vi"("pos"=w633, "exist"=w634, "available"=w635, "redTurn"=w636) -> ("availableNew"=w637:i32[][])  [unwired: 4 in, 3 out]
                        n496 = local write "availables"(w637) -> ()
                      }
                      frame #1 {
                        n497 = local read "pressedI"() -> (w639:i32)
                        n498 = local read "pressedJ"() -> (w638:i32)
                        n499 = local read "availables"() -> (w641:i32[][])
                        n500 = Add(x=w639, y=w638) -> (x+y=w642:i32)
                        n501 = Greater Or Equal To 0?(x=w642) -> (x >= 0?=w640:bool)
                        n502 = case shown="True" w640 {
                          tunnel: w641 -> [_ w647]
                          tunnel: w639 -> [_ w646]
                          tunnel: w638 -> [_ w645]
                          frame False {
                          }
                          frame True {
                            n503 = Index Array(array=w647, index (row)=w646, index (col)=w645) -> (element=w643:i32)
                            n504 = Greater Than 0?(x=w643) -> (x > 0?=w644:bool)
                            n505 = case shown="True" w644 {
                              frame False {
                                # "error mess."
                                n506 = disable-structure shown="Disabled" {
                                frame Disabled {
                                n507 = local read "Turn"() -> (w650:i32)
                                n508 = Subtract(x=1 ("y"), y=w650) -> (x-y=w648:i32)
                                n509 = local write "Turn"(w648) -> ()
                                }
                                frame Enabled {
                                }
                                }
                                n510 = call "Display Message to User9"() -> ()  [unwired: 10 in, 2 out]
                              }
                              frame True {
                                n511 = stacked-sequence {
                                frame #0 {
                                n512 = local read "currentState.exist"() -> (w656:i32[][])
                                n513 = local read "currentState.pos"() -> (w655:i32[][])
                                n514 = local read "pressedJ"() -> (w651:i32)
                                n515 = local read "pressedI"() -> (w652:i32)
                                n516 = local read "Turn"() -> (w657:i32)
                                n517 = call "takeStep.vi"("redTurn"=w657, "pos"=w655, "exist"=w656, "j"=w651, "i"=w652) -> ("posNew"=w653:i32[][], "existNew"=w654:i32[][])  [unwired: 4 in, 1 out]
                                n518 = local write "currentState.exist"(w654) -> ()
                                n519 = local write "currentState.pos"(w653) -> ()
                                }
                                frame #1 {
                                # "下完後要準備將資料上傳"
                                n520 = local write "putToNet"(TRUE ("getFromNet")) -> ()
                                }
                                frame #2 {
                                # "換人下"
                                n521 = local read "Turn"() -> (w661:i32)
                                n522 = Subtract(x=1 ("y"), y=w661) -> (x-y=w659:i32)
                                n523 = local write "Turn"(w659) -> ()
                                }
                                frame #3 {
                                n524 = local read "currentState.exist"() -> (w664:i32[][])
                                n525 = local read "currentState.pos"() -> (w663:i32[][])
                                n526 = local read "availables"() -> (w665:i32[][])
                                n527 = local read "Turn"() -> (w666:i32)
                                n528 = call "availablePlaces.vi"("pos"=w663, "exist"=w664, "available"=w665, "redTurn"=w666) -> ("posNew"=w669:i32[][], "existNew"=w668:i32[][], "availableNew"=w667:i32[][], "count"=w670:i32)  [unwired: 4 in]
                                n529 = local write "currentState.exist"(w668) -> ()
                                n530 = local write "currentState.pos"(w669) -> ()
                                n531 = local write "availables"(w667) -> ()
                                n532 = Equal To 0?(x=w670) -> (x = 0?=w662:bool)
                                n533 = case shown="True" w662 {
                                frame False {
                                }
                                frame True {
                                n534 = local read "Turn"() -> (w672:i32)
                                n535 = Subtract(x=1 ("y"), y=w672) -> (x-y=w671:i32)
                                n536 = local write "Turn"(w671) -> ()
                                }
                                }
                                }
                                frame #4 {
                                n537 = local read "currentState.exist"() -> (w675:i32[][])
                                n538 = local read "currentState.pos"() -> (w676:i32[][])
                                n539 = call "countResult.vi"("pos"=w676, "exist"=w675) -> ("result"=w674:i32)  [unwired: 9 in]
                                n540 = local write "result"(w674) -> ()
                                }
                                }
                              }
                            }
                          }
                        }
                      }
                    }
                  }
                  frame #1 {
                    n541 = local read "currentState.exist"() -> (w679:i32[][])
                    n542 = local read "currentState.pos"() -> (w678:i32[][])
                    n543 = call "isEnd.vi"("pos"=w678, "exist"=w679) -> ("isEnd"=w677:i16)  [unwired: 9 in]
                    n544 = case shown="1" w677 {
                      frame 0, Default {
                      }
                      frame 1 {
                        # "gameover"
                        n545 = flat-sequence {
                          frame #0 {
                            n546 = local read "result"() -> (w688:i32)
                            n547 = Greater Than 0?(x=w688) -> (x > 0?=w686:bool)
                            n548 = Select(t="Black win ", s=w686, f="White win ") -> (s? t:f=w687:string)
                            n549 = Absolute Value(x=w688) -> (abs(x)=w689:i32)
                            n550 = Number To Decimal String(number=w689) -> (decimal integer string=w690:string)  [unwired: 1 in]
                            n551 = Concatenate Strings("GAME OVER", "\r\n", w687, w690, " points" ("string")) -> (w682:string)
                            n552 = call "Display Message to User10"("Message"=w682) -> ()  [unwired: 9 in, 2 out]
                          }
                          frame #1 {
                            n553 = local write "GameOver"(TRUE ("PowerOff")) -> ()
                          }
                        }
                      }
                    }
                  }
                  frame #2 {
                    n554 = flat-sequence {
                      frame #0 {
                        # "將資料放到網路上後準備接收資料"
                        n555 = local read "putToNet"() -> (w692:bool)
                        n556 = case shown="True" w692 {
                          frame False {
                          }
                          frame True {
                            n557 = flat-sequence {
                              frame #0 {
                                w697 = -1000 ("pressedJ")
                                n558 = local read "currentState.exist"() -> (w695:i32[][])
                                n559 = local read "currentState.pos"() -> (w694:i32[][])
                                n560 = local write "pressedI"(w697) -> ()
                                n561 = local write "pressedJ"(w697) -> ()
                                n562 = for {
                                tunnel: w695 -> [w700] mode=indexing
                                tunnel: w694 -> [w699] mode=indexing
                                tunnel: [w698] -> w696 mode=indexing
                                n563 = for {
                                tunnel: w700 -> [w703] mode=indexing
                                tunnel: w699 -> [w702] mode=indexing
                                tunnel: [w701] -> w698 mode=indexing
                                n564 = Add(x=w703, y=w702) -> (x+y=w701:i32)
                                }
                                }
                                n565 = local write "getFromNet"(TRUE) -> ()
                                n566 = call "server.vi"("array"=w696) -> ()  [unwired: 10 in, 1 out]
                              }
                              frame #1 {
                                n567 = local write "putToNet"(FALSE) -> ()
                              }
                            }
                          }
                        }
                      }
                      frame #1 {
                        n568 = local read "getFromNet"() -> (w705:bool)
                        n569 = case shown="True" w705 {
                          frame False {
                          }
                          frame True {
                            n570 = flat-sequence {
                              frame #0 {
                                # "接收資料後將其還原"
                                n571 = call "client.vi"() -> ("value"=w707:i32[][])  [unwired: 10 in, 1 out]
                                n572 = for {
                                tunnel: w707 -> [w710] mode=indexing
                                tunnel: [w708] -> w706 mode=indexing
                                i -> [w709]
                                n573 = for {
                                tunnel: w710 -> [w712] mode=indexing
                                tunnel: w709 -> [w714]
                                tunnel: [w711] -> w708 mode=indexing
                                i -> [w713]
                                n574 = Greater?(x=w712, y=0) -> (0:w715:bool)
                                n575 = case shown="True" w715 {
                                tunnel: w714 -> [_ w722]
                                tunnel: w713 -> [_ w721]
                                tunnel: [w717 w719] -> w711
                                tunnel: w712 -> [w717 w718]
                                frame False {
                                }
                                frame True {
                                n576 = local read "currentState.exist"() -> (w723:i32[][])
                                n577 = Replace Array Subset(array=w723, new element=1 ("new element/subarray"), index (row)=w722, index (col)=w721) -> (w724:i32[][])
                                n578 = Decrement(x=w718) -> (x-1=w719:i32)
                                n579 = local write "currentState.exist"(w724) -> ()
                                }
                                }
                                }
                                }
                                n580 = local write "currentState.pos"(w706) -> ()
                              }
                              frame #1 {
                                n581 = local write "getFromNet"(FALSE ("getFromNet")) -> ()
                                n582 = local write "Turn"(0 ("redTurn")) -> ()
                                n583 = local write "Turn"(i8 0 ("redTurn")) -> ()
                              }
                            }
                          }
                        }
                      }
                    }
                  }
                  frame #3 {
                    # "下載資料後更新可下的點"
                    n584 = local read "currentState.exist"() -> (w729:i32[][])
                    n585 = local read "currentState.pos"() -> (w728:i32[][])
                    n586 = local read "availables"() -> (w730:i32[][])
                    n587 = local read "Turn"() -> (w731:i32)
                    n588 = call "availablePlaces.vi"("pos"=w728, "exist"=w729, "available"=w730, "redTurn"=w731) -> ("availableNew"=w732:i32[][])  [unwired: 4 in, 3 out]
                    n589 = local write "availables"(w732) -> ()
                  }
                }
              }
              frame Default {
                # "各模式初始化"
                # "模式代碼"
                # "模式選擇:每個按鈕按會對應不同模式代碼"
                n590 = event shown="[0] Timeout" {
                  selector: _ -> [_ _ _ _ _ _ _]
                  dyn-events: _ -> [_ _ _ _ _ _ _]
                  timeout: 100 -> [_ _ _ _ _ _ _]
                  tunnel: [0 ("difficulty") -33121260 ("y") 21414112 ("y") w764 3422134 ("x") 4312243 ("x") 19735 ("x")] -> w733
                  event Timeout {
                    n591 = event-data() -> ()  [unwired: 1 in, 3 out]
                  }
                  event "PVP": Mouse Down {
                    n592 = event-data() -> ()  [unwired: 1 in, 8 out]
                  }
                  event "EVE": Mouse Down {
                    n593 = event-data() -> ()  [unwired: 1 in, 8 out]
                  }
                  event "PVE": Mouse Down {
                    n594 = event-data() -> ()  [unwired: 1 in, 8 out]
                    n595 = call "Prompt User for Input"() -> ("difficulty"=w765:dbl)  [unwired: 17 in, 2 out]
                    n596 = To Long Integer(number=w765) -> (32bit integer=w764:i32)
                  }
                  event "OL(host,black)": Mouse Down {
                    n597 = event-data() -> ()  [unwired: 1 in, 8 out]
                  }
                  event "OL(client,white)": Mouse Down {
                    n598 = event-data() -> ()  [unwired: 1 in, 8 out]
                    n599 = local write "getFromNet"(TRUE ("getFromNet")) -> ()
                  }
                  event "OL(continue)": Mouse Down {
                    n600 = event-data() -> ()  [unwired: 1 in, 8 out]
                    n601 = local write "getFromNet"(TRUE ("getFromNet")) -> ()
                  }
                }
                n602 = case shown="Default" w733 {
                  tunnel: [TRUE TRUE TRUE FALSE TRUE TRUE TRUE TRUE TRUE] -> w736
                  tunnel: ["online white" ("mode 2") "online black" ("mode 2") w742 "Home" ("mode 2") "easy" ("mode 2") "normal" ("mode 2") "hard" ("mode 2") "2players" ("mode 2") "AI" ("mode 2")] -> w735
                  frame 4312243 {
                  }
                  frame 3422134 {
                  }
                  frame 19735 {
                    n603 = call "Prompt User for Input2"() -> ("white"=w743:bool)  [unwired: 18 in, 1 out]
                    n604 = case shown="True" w743 {
                      tunnel: ["online balck" ("mode 2") "online white" ("mode 2")] -> w742
                      tunnel: [1 0] -> w741
                      frame False {
                      }
                      frame True {
                      }
                    }
                    n605 = local write "Turn"(w741) -> ()
                  }
                  frame Default {
                  }
                  frame 1 {
                  }
                  frame 2 {
                  }
                  frame 3 {
                  }
                  frame -33121260 {
                  }
                  frame 21414112 {
                  }
                }
                "mode" <- w735
                n606 = local write "mode/difficulty"(w733) -> ()
                n607 = property on="mode" class="Str"("Visible"=w736) -> ()  [unwired: 2 in, 2 out]
              }
            }
          }
        }
      }
      n608 = while {
        stop <- w151 stop-if-true
        w106 = 7 ("index (row)")
        w105 = 6 ("index (row)")
        w88 = 5 ("index (row)")
        w87 = 4 ("index (row)")
        w123 = 3 ("index (row)")
        w124 = 2 ("index (row)")
        w141 = 1 ("index (row)")
        w142 = 0 ("index (row)")
        # "將接下來可以下的位置以特殊顏色標示"
        # "Display availiable places"
        n609 = local read "availables"() -> (w17:i32[][])
        n610 = call "canBePlaced.vi"("array"=w17, "index (col)"=4 ("disabled index (col)"), "index (row)"=w142) -> ("color"=w75:cluster{u32, u32}[])  [unwired: 8 in]
        n611 = call "canBePlaced.vi"("array"=w17, "index (col)"=3 ("disabled index (col)"), "index (row)"=w142) -> ("color"=w76:cluster{u32, u32}[])  [unwired: 8 in]
        n612 = call "canBePlaced.vi"("array"=w17, "index (col)"=7 ("disabled index (col)"), "index (row)"=w142) -> ("color"=w72:cluster{u32, u32}[])  [unwired: 8 in]
        n613 = call "canBePlaced.vi"("array"=w17, "index (col)"=5 ("disabled index (col)"), "index (row)"=w142) -> ("color"=w74:cluster{u32, u32}[])  [unwired: 8 in]
        n614 = call "canBePlaced.vi"("array"=w17, "index (col)"=6 ("disabled index (col)"), "index (row)"=w142) -> ("color"=w73:cluster{u32, u32}[])  [unwired: 8 in]
        n615 = call "canBePlaced.vi"("array"=w17, "index (col)"=1 ("disabled index (col)"), "index (row)"=w142) -> ("color"=w78:cluster{u32, u32}[])  [unwired: 8 in]
        n616 = call "canBePlaced.vi"("array"=w17, "index (col)"=2 ("disabled index (col)"), "index (row)"=w142) -> ("color"=w77:cluster{u32, u32}[])  [unwired: 8 in]
        n617 = call "canBePlaced.vi"("array"=w17, "index (col)"=0 ("disabled index (col)"), "index (row)"=w142) -> ("color"=w149:cluster{u32, u32}[])  [unwired: 8 in]
        n618 = property on="0 3" class="Bool (strict)"("Colors [4]"=w76) -> ()  [unwired: 2 in, 2 out]
        n619 = property on="0 6" class="Bool (strict)"("Colors [4]"=w73) -> ()  [unwired: 2 in, 2 out]
        n620 = property on="0 7" class="Bool (strict)"("Colors [4]"=w72) -> ()  [unwired: 2 in, 2 out]
        n621 = property on="0 4" class="Bool (strict)"("Colors [4]"=w75) -> ()  [unwired: 2 in, 2 out]
        n622 = property on="0 5" class="Bool (strict)"("Colors [4]"=w74) -> ()  [unwired: 2 in, 2 out]
        n623 = property on="0 2" class="Bool (strict)"("Colors [4]"=w77) -> ()  [unwired: 2 in, 2 out]
        n624 = property on="0 1" class="Bool (strict)"("Colors [4]"=w78) -> ()  [unwired: 2 in, 2 out]
        n625 = property on="0 0" class="Bool (strict)"("Colors [4]"=w149) -> ()  [unwired: 2 in, 2 out]
        n626 = call "canBePlaced.vi"("array"=w17, "index (col)"=4 ("disabled index (col)"), "index (row)"=w141) -> ("color"=w66:cluster{u32, u32}[])  [unwired: 8 in]
        n627 = call "canBePlaced.vi"("array"=w17, "index (col)"=3 ("disabled index (col)"), "index (row)"=w141) -> ("color"=w67:cluster{u32, u32}[])  [unwired: 8 in]
        n628 = call "canBePlaced.vi"("array"=w17, "index (col)"=7 ("disabled index (col)"), "index (row)"=w141) -> ("color"=w63:cluster{u32, u32}[])  [unwired: 8 in]
        n629 = call "canBePlaced.vi"("array"=w17, "index (col)"=5 ("disabled index (col)"), "index (row)"=w141) -> ("color"=w65:cluster{u32, u32}[])  [unwired: 8 in]
        n630 = call "canBePlaced.vi"("array"=w17, "index (col)"=6 ("disabled index (col)"), "index (row)"=w141) -> ("color"=w64:cluster{u32, u32}[])  [unwired: 8 in]
        n631 = call "canBePlaced.vi"("array"=w17, "index (col)"=1 ("disabled index (col)"), "index (row)"=w141) -> ("color"=w69:cluster{u32, u32}[])  [unwired: 8 in]
        n632 = call "canBePlaced.vi"("array"=w17, "index (col)"=2 ("disabled index (col)"), "index (row)"=w141) -> ("color"=w68:cluster{u32, u32}[])  [unwired: 8 in]
        n633 = call "canBePlaced.vi"("array"=w17, "index (col)"=0 ("disabled index (col)"), "index (row)"=w141) -> ("color"=w70:cluster{u32, u32}[])  [unwired: 8 in]
        n634 = property on="1 7" class="Bool (strict)"("Colors [4]"=w63) -> ()  [unwired: 2 in, 2 out]
        n635 = property on="1 3" class="Bool (strict)"("Colors [4]"=w67) -> ()  [unwired: 2 in, 2 out]
        n636 = property on="1 6" class="Bool (strict)"("Colors [4]"=w64) -> ()  [unwired: 2 in, 2 out]
        n637 = property on="1 4" class="Bool (strict)"("Colors [4]"=w66) -> ()  [unwired: 2 in, 2 out]
        n638 = property on="1 5" class="Bool (strict)"("Colors [4]"=w65) -> ()  [unwired: 2 in, 2 out]
        n639 = property on="1 2" class="Bool (strict)"("Colors [4]"=w68) -> ()  [unwired: 2 in, 2 out]
        n640 = property on="1 0" class="Bool (strict)"("Colors [4]"=w70) -> ()  [unwired: 2 in, 2 out]
        n641 = property on="1 1" class="Bool (strict)"("Colors [4]"=w69) -> ()  [unwired: 2 in, 2 out]
        n642 = call "canBePlaced.vi"("array"=w17, "index (col)"=4 ("disabled index (col)"), "index (row)"=w124) -> ("color"=w59:cluster{u32, u32}[])  [unwired: 8 in]
        n643 = call "canBePlaced.vi"("array"=w17, "index (col)"=3 ("disabled index (col)"), "index (row)"=w124) -> ("color"=w60:cluster{u32, u32}[])  [unwired: 8 in]
        n644 = call "canBePlaced.vi"("array"=w17, "index (col)"=7 ("disabled index (col)"), "index (row)"=w124) -> ("color"=w56:cluster{u32, u32}[])  [unwired: 8 in]
        n645 = call "canBePlaced.vi"("array"=w17, "index (col)"=5 ("disabled index (col)"), "index (row)"=w124) -> ("color"=w58:cluster{u32, u32}[])  [unwired: 8 in]
        n646 = call "canBePlaced.vi"("array"=w17, "index (col)"=6 ("disabled index (col)"), "index (row)"=w124) -> ("color"=w57:cluster{u32, u32}[])  [unwired: 8 in]
        n647 = call "canBePlaced.vi"("array"=w17, "index (col)"=1 ("disabled index (col)"), "index (row)"=w124) -> ("color"=w62:cluster{u32, u32}[])  [unwired: 8 in]
        n648 = call "canBePlaced.vi"("array"=w17, "index (col)"=2 ("disabled index (col)"), "index (row)"=w124) -> ("color"=w61:cluster{u32, u32}[])  [unwired: 8 in]
        n649 = call "canBePlaced.vi"("array"=w17, "index (col)"=0 ("disabled index (col)"), "index (row)"=w124) -> ("color"=w71:cluster{u32, u32}[])  [unwired: 8 in]
        n650 = property on="2 7" class="Bool (strict)"("Colors [4]"=w56) -> ()  [unwired: 2 in, 2 out]
        n651 = property on="2 5" class="Bool (strict)"("Colors [4]"=w58) -> ()  [unwired: 2 in, 2 out]
        n652 = property on="2 6" class="Bool (strict)"("Colors [4]"=w57) -> ()  [unwired: 2 in, 2 out]
        n653 = property on="2 1" class="Bool (strict)"("Colors [4]"=w62) -> ()  [unwired: 2 in, 2 out]
        n654 = property on="2 2" class="Bool (strict)"("Colors [4]"=w61) -> ()  [unwired: 2 in, 2 out]
        n655 = property on="2 4" class="Bool (strict)"("Colors [4]"=w59) -> ()  [unwired: 2 in, 2 out]
        n656 = property on="2 3" class="Bool (strict)"("Colors [4]"=w60) -> ()  [unwired: 2 in, 2 out]
        n657 = property on="2 0" class="Bool (strict)"("Colors [4]"=w71) -> ()  [unwired: 2 in, 2 out]
        n658 = local read "PowerOff"() -> (w151:bool)
        n659 = call "canBePlaced.vi"("array"=w17, "index (col)"=4 ("disabled index (col)"), "index (row)"=w123) -> ("color"=w51:cluster{u32, u32}[])  [unwired: 8 in]
        n660 = call "canBePlaced.vi"("array"=w17, "index (col)"=3 ("disabled index (col)"), "index (row)"=w123) -> ("color"=w52:cluster{u32, u32}[])  [unwired: 8 in]
        n661 = call "canBePlaced.vi"("array"=w17, "index (col)"=7 ("disabled index (col)"), "index (row)"=w123) -> ("color"=w48:cluster{u32, u32}[])  [unwired: 8 in]
        n662 = call "canBePlaced.vi"("array"=w17, "index (col)"=5 ("disabled index (col)"), "index (row)"=w123) -> ("color"=w50:cluster{u32, u32}[])  [unwired: 8 in]
        n663 = call "canBePlaced.vi"("array"=w17, "index (col)"=6 ("disabled index (col)"), "index (row)"=w123) -> ("color"=w49:cluster{u32, u32}[])  [unwired: 8 in]
        n664 = call "canBePlaced.vi"("array"=w17, "index (col)"=1 ("disabled index (col)"), "index (row)"=w123) -> ("color"=w54:cluster{u32, u32}[])  [unwired: 8 in]
        n665 = call "canBePlaced.vi"("array"=w17, "index (col)"=2 ("disabled index (col)"), "index (row)"=w123) -> ("color"=w53:cluster{u32, u32}[])  [unwired: 8 in]
        n666 = call "canBePlaced.vi"("array"=w17, "index (col)"=0 ("disabled index (col)"), "index (row)"=w123) -> ("color"=w55:cluster{u32, u32}[])  [unwired: 8 in]
        n667 = property on="3 4" class="Bool (strict)"("Colors [4]"=w51) -> ()  [unwired: 2 in, 2 out]
        n668 = property on="3 5" class="Bool (strict)"("Colors [4]"=w50) -> ()  [unwired: 2 in, 2 out]
        n669 = property on="3 7" class="Bool (strict)"("Colors [4]"=w48) -> ()  [unwired: 2 in, 2 out]
        n670 = property on="3 3" class="Bool (strict)"("Colors [4]"=w52) -> ()  [unwired: 2 in, 2 out]
        n671 = property on="3 1" class="Bool (strict)"("Colors [4]"=w54) -> ()  [unwired: 2 in, 2 out]
        n672 = property on="3 0" class="Bool (strict)"("Colors [4]"=w55) -> ()  [unwired: 2 in, 2 out]
        n673 = property on="3 2" class="Bool (strict)"("Colors [4]"=w53) -> ()  [unwired: 2 in, 2 out]
        n674 = property on="3 6" class="Bool (strict)"("Colors [4]"=w49) -> ()  [unwired: 2 in, 2 out]
        n675 = call "canBePlaced.vi"("array"=w17, "index (col)"=4 ("disabled index (col)"), "index (row)"=w87) -> ("color"=w44:cluster{u32, u32}[])  [unwired: 8 in]
        n676 = call "canBePlaced.vi"("array"=w17, "index (col)"=3 ("disabled index (col)"), "index (row)"=w87) -> ("color"=w43:cluster{u32, u32}[])  [unwired: 8 in]
        n677 = call "canBePlaced.vi"("array"=w17, "index (col)"=7 ("disabled index (col)"), "index (row)"=w87) -> ("color"=w47:cluster{u32, u32}[])  [unwired: 8 in]
        n678 = call "canBePlaced.vi"("array"=w17, "index (col)"=5 ("disabled index (col)"), "index (row)"=w87) -> ("color"=w45:cluster{u32, u32}[])  [unwired: 8 in]
        n679 = call "canBePlaced.vi"("array"=w17, "index (col)"=6 ("disabled index (col)"), "index (row)"=w87) -> ("color"=w46:cluster{u32, u32}[])  [unwired: 8 in]
        n680 = call "canBePlaced.vi"("array"=w17, "index (col)"=1 ("disabled index (col)"), "index (row)"=w87) -> ("color"=w20:cluster{u32, u32}[])  [unwired: 8 in]
        n681 = call "canBePlaced.vi"("array"=w17, "index (col)"=2 ("disabled index (col)"), "index (row)"=w87) -> ("color"=w42:cluster{u32, u32}[])  [unwired: 8 in]
        n682 = call "canBePlaced.vi"("array"=w17, "index (col)"=0 ("disabled index (col)"), "index (row)"=w87) -> ("color"=w41:cluster{u32, u32}[])  [unwired: 8 in]
        n683 = property on="4 1" class="Bool (strict)"("Colors [4]"=w20) -> ()  [unwired: 2 in, 2 out]
        n684 = property on="4 2" class="Bool (strict)"("Colors [4]"=w42) -> ()  [unwired: 2 in, 2 out]
        n685 = property on="4 3" class="Bool (strict)"("Colors [4]"=w43) -> ()  [unwired: 2 in, 2 out]
        n686 = property on="4 5" class="Bool (strict)"("Colors [4]"=w45) -> ()  [unwired: 2 in, 2 out]
        n687 = property on="4 7" class="Bool (strict)"("Colors [4]"=w47) -> ()  [unwired: 2 in, 2 out]
        n688 = property on="4 4" class="Bool (strict)"("Colors [4]"=w44) -> ()  [unwired: 2 in, 2 out]
        n689 = property on="4 0" class="Bool (strict)"("Colors [4]"=w41) -> ()  [unwired: 2 in, 2 out]
        n690 = property on="4 6" class="Bool (strict)"("Colors [4]"=w46) -> ()  [unwired: 2 in, 2 out]
        n691 = call "canBePlaced.vi"("array"=w17, "index (col)"=4 ("disabled index (col)"), "index (row)"=w88) -> ("color"=w37:cluster{u32, u32}[])  [unwired: 8 in]
        n692 = call "canBePlaced.vi"("array"=w17, "index (col)"=3 ("disabled index (col)"), "index (row)"=w88) -> ("color"=w38:cluster{u32, u32}[])  [unwired: 8 in]
        n693 = call "canBePlaced.vi"("array"=w17, "index (col)"=7 ("disabled index (col)"), "index (row)"=w88) -> ("color"=w34:cluster{u32, u32}[])  [unwired: 8 in]
        n694 = call "canBePlaced.vi"("array"=w17, "index (col)"=5 ("disabled index (col)"), "index (row)"=w88) -> ("color"=w36:cluster{u32, u32}[])  [unwired: 8 in]
        n695 = call "canBePlaced.vi"("array"=w17, "index (col)"=6 ("disabled index (col)"), "index (row)"=w88) -> ("color"=w35:cluster{u32, u32}[])  [unwired: 8 in]
        n696 = call "canBePlaced.vi"("array"=w17, "index (col)"=1 ("disabled index (col)"), "index (row)"=w88) -> ("color"=w40:cluster{u32, u32}[])  [unwired: 8 in]
        n697 = call "canBePlaced.vi"("array"=w17, "index (col)"=2 ("disabled index (col)"), "index (row)"=w88) -> ("color"=w39:cluster{u32, u32}[])  [unwired: 8 in]
        n698 = call "canBePlaced.vi"("array"=w17, "index (col)"=0 ("disabled index (col)"), "index (row)"=w88) -> ("color"=w19:cluster{u32, u32}[])  [unwired: 8 in]
        n699 = property on="5 7" class="Bool (strict)"("Colors [4]"=w34) -> ()  [unwired: 2 in, 2 out]
        n700 = property on="5 4" class="Bool (strict)"("Colors [4]"=w37) -> ()  [unwired: 2 in, 2 out]
        n701 = property on="5 1" class="Bool (strict)"("Colors [4]"=w40) -> ()  [unwired: 2 in, 2 out]
        n702 = property on="5 3" class="Bool (strict)"("Colors [4]"=w38) -> ()  [unwired: 2 in, 2 out]
        n703 = property on="5 5" class="Bool (strict)"("Colors [4]"=w36) -> ()  [unwired: 2 in, 2 out]
        n704 = property on="5 6" class="Bool (strict)"("Colors [4]"=w35) -> ()  [unwired: 2 in, 2 out]
        n705 = property on="5 2" class="Bool (strict)"("Colors [4]"=w39) -> ()  [unwired: 2 in, 2 out]
        n706 = property on="5 0" class="Bool (strict)"("Colors [4]"=w19) -> ()  [unwired: 2 in, 2 out]
        n707 = call "canBePlaced.vi"("array"=w17, "index (col)"=4 ("disabled index (col)"), "index (row)"=w105) -> ("color"=w29:cluster{u32, u32}[])  [unwired: 8 in]
        n708 = call "canBePlaced.vi"("array"=w17, "index (col)"=3 ("disabled index (col)"), "index (row)"=w105) -> ("color"=w30:cluster{u32, u32}[])  [unwired: 8 in]
        n709 = call "canBePlaced.vi"("array"=w17, "index (col)"=7 ("disabled index (col)"), "index (row)"=w105) -> ("color"=w26:cluster{u32, u32}[])  [unwired: 8 in]
        n710 = call "canBePlaced.vi"("array"=w17, "index (col)"=5 ("disabled index (col)"), "index (row)"=w105) -> ("color"=w28:cluster{u32, u32}[])  [unwired: 8 in]
        n711 = call "canBePlaced.vi"("array"=w17, "index (col)"=6 ("disabled index (col)"), "index (row)"=w105) -> ("color"=w27:cluster{u32, u32}[])  [unwired: 8 in]
        n712 = call "canBePlaced.vi"("array"=w17, "index (col)"=1 ("disabled index (col)"), "index (row)"=w105) -> ("color"=w32:cluster{u32, u32}[])  [unwired: 8 in]
        n713 = call "canBePlaced.vi"("array"=w17, "index (col)"=2 ("disabled index (col)"), "index (row)"=w105) -> ("color"=w31:cluster{u32, u32}[])  [unwired: 8 in]
        n714 = call "canBePlaced.vi"("array"=w17, "index (col)"=0 ("disabled index (col)"), "index (row)"=w105) -> ("color"=w33:cluster{u32, u32}[])  [unwired: 8 in]
        n715 = property on="6 5" class="Bool (strict)"("Colors [4]"=w28) -> ()  [unwired: 2 in, 2 out]
        n716 = property on="6 7" class="Bool (strict)"("Colors [4]"=w26) -> ()  [unwired: 2 in, 2 out]
        n717 = property on="6 4" class="Bool (strict)"("Colors [4]"=w29) -> ()  [unwired: 2 in, 2 out]
        n718 = property on="6 3" class="Bool (strict)"("Colors [4]"=w30) -> ()  [unwired: 2 in, 2 out]
        n719 = property on="6 1" class="Bool (strict)"("Colors [4]"=w32) -> ()  [unwired: 2 in, 2 out]
        n720 = property on="6 2" class="Bool (strict)"("Colors [4]"=w31) -> ()  [unwired: 2 in, 2 out]
        n721 = property on="6 6" class="Bool (strict)"("Colors [4]"=w27) -> ()  [unwired: 2 in, 2 out]
        n722 = property on="6 0" class="Bool (strict)"("Colors [4]"=w33) -> ()  [unwired: 2 in, 2 out]
        n723 = call "canBePlaced.vi"("array"=w17, "index (col)"=4 ("disabled index (col)"), "index (row)"=w106) -> ("color"=w16:cluster{u32, u32}[])  [unwired: 8 in]
        n724 = call "canBePlaced.vi"("array"=w17, "index (col)"=3 ("disabled index (col)"), "index (row)"=w106) -> ("color"=w24:cluster{u32, u32}[])  [unwired: 8 in]
        n725 = call "canBePlaced.vi"("array"=w17, "index (col)"=7 ("disabled index (col)"), "index (row)"=w106) -> ("color"=w21:cluster{u32, u32}[])  [unwired: 8 in]
        n726 = call "canBePlaced.vi"("array"=w17, "index (col)"=5 ("disabled index (col)"), "index (row)"=w106) -> ("color"=w23:cluster{u32, u32}[])  [unwired: 8 in]
        n727 = call "canBePlaced.vi"("array"=w17, "index (col)"=6 ("disabled index (col)"), "index (row)"=w106) -> ("color"=w22:cluster{u32, u32}[])  [unwired: 8 in]
        n728 = call "canBePlaced.vi"("array"=w17, "index (col)"=1 ("disabled index (col)"), "index (row)"=w106) -> ("color"=w15:cluster{u32, u32}[])  [unwired: 8 in]
        n729 = call "canBePlaced.vi"("array"=w17, "index (col)"=2 ("disabled index (col)"), "index (row)"=w106) -> ("color"=w18:cluster{u32, u32}[])  [unwired: 8 in]
        n730 = call "canBePlaced.vi"("array"=w17, "index (col)"=0 ("disabled index (col)"), "index (row)"=w106) -> ("color"=w25:cluster{u32, u32}[])  [unwired: 8 in]
        n731 = property on="7 5" class="Bool (strict)"("Colors [4]"=w23) -> ()  [unwired: 2 in, 2 out]
        n732 = property on="7 6" class="Bool (strict)"("Colors [4]"=w22) -> ()  [unwired: 2 in, 2 out]
        n733 = property on="7 7" class="Bool (strict)"("Colors [4]"=w21) -> ()  [unwired: 2 in, 2 out]
        n734 = property on="7 4" class="Bool (strict)"("Colors [4]"=w16) -> ()  [unwired: 2 in, 2 out]
        n735 = property on="7 3" class="Bool (strict)"("Colors [4]"=w24) -> ()  [unwired: 2 in, 2 out]
        n736 = property on="7 0" class="Bool (strict)"("Colors [4]"=w25) -> ()  [unwired: 2 in, 2 out]
        n737 = property on="7 1" class="Bool (strict)"("Colors [4]"=w15) -> ()  [unwired: 2 in, 2 out]
        n738 = property on="7 2" class="Bool (strict)"("Colors [4]"=w18) -> ()  [unwired: 2 in, 2 out]
        n739 = Wait Until Next ms Multiple(millisecond multiple=u32 200) -> ()  [unwired: 1 out]
      }
      n740 = call "initialize(picture).vi"("picture size"=w11) -> ("2D Picture"=w12:picture)  [unwired: 10 in]
      n741 = while {
        shift-right: [w778] -> _
        shift-left: w12 -> [w782]
        tunnel: w11 -> [w777]
        i -> [w773]
        stop <- w774 stop-if-true
        # "檢查棋盤上的值，並更新圖上黑白子顯示"
        # "被按之按鈕座標(若無按按鈕則皆為-1000)"
        # "按按鈕的反應啟動(每個按鈕對應棋盤上一處)"
        # "棋盤顯示"
        n742 = event shown="[0] Timeout" {
          selector: _ -> [_ _ _ _ _ _ _ _ _ _ _ _ _ _ _ _ _ _ _ _ _ _ _ _ _ _ _ _ _ _ _ _ _ _ _ _ _ _ _ _ _ _ _ _ _ _ _ _ _ _ _ _ _ _ _ _ _ _ _ _ _ _ _ _ _]
          dyn-events: _ -> [_ _ _ _ _ _ _ _ _ _ _ _ _ _ _ _ _ _ _ _ _ _ _ _ _ _ _ _ _ _ _ _ _ _ _ _ _ _ _ _ _ _ _ _ _ _ _ _ _ _ _ _ _ _ _ _ _ _ _ _ _ _ _ _ _]
          timeout: 100 -> [_ _ _ _ _ _ _ _ _ _ _ _ _ _ _ _ _ _ _ _ _ _ _ _ _ _ _ _ _ _ _ _ _ _ _ _ _ _ _ _ _ _ _ _ _ _ _ _ _ _ _ _ _ _ _ _ _ _ _ _ _ _ _ _ _]
          tunnel: [w812 w815 w818 w821 w824 w827 w830 w833 w836 w839 w842 w845 w848 w851 w854 w857 w860 w863 w866 w869 w872 w875 w878 w881 w884 w887 w890 w893 w896 w899 w902 w905 w908 w911 w914 w917 w920 w923 w926 w929 w932 w935 w938 w941 w944 w947 w950 w953 w956 w959 w962 w965 w968 w971 w974 w977 w980 w983 w986 w989 w992 w995 w998 w1001 w1004] -> w779
          tunnel: w782 -> [w812 w815 w818 w821 w824 w827 w830 w833 w836 w839 w842 w845 w848 w851 w854 w857 w860 w863 w866 w869 w872 w875 w878 w881 w884 w887 w890 w893 w896 w899 w902 w905 w908 w911 w914 w917 w920 w923 w926 w929 w932 w935 w938 w941 w944 w947 w950 w953 w956 w959 w962 w965 w968 w971 w974 w977 w980 w983 w986 w989 w992 w995 w998 w1001 w1004]
          tunnel: [-1000 ("index (row)") 0 ("index (row)") 0 ("index (row)") 0 ("index (row)") 0 ("index (row)") 0 ("index (row)") 0 ("index (row)") 0 ("index (row)") 0 ("index (row)") 1 ("index (row)") 1 ("index (row)") 1 ("index (row)") 1 ("index (row)") 1 ("index (row)") 1 ("index (row)") 1 ("index (row)") 1 ("index (row)") 2 ("index (row)") 2 ("index (row)") 2 ("index (row)") 2 ("index (row)") 2 ("index (row)") 2 ("index (row)") 2 ("index (row)") 2 ("index (row)") 3 ("index (row)") 3 ("index (row)") 3 ("index (row)") 3 ("index (row)") 3 ("index (row)") 3 ("index (row)") 3 ("index (row)") 3 ("index (row)") 4 ("index (row)") 4 ("index (row)") 4 ("index (row)") 4 ("index (row)") 4 ("index (row)") 4 ("index (row)") 4 ("index (row)") 4 ("index (row)") 5 ("index (row)") 5 ("index (row)") 5 ("index (row)") 5 ("index (row)") 5 ("index (row)") 5 ("index (row)") 5 ("index (row)") 5 ("index (row)") 6 ("index (row)") 6 ("index (row)") 6 ("index (row)") 6 ("index (row)") 6 ("index (row)") 6 ("index (row)") 6 ("index (row)") 6 ("index (row)") 7 ("index (row)") 7 ("index (row)") 7 ("index (row)") 7 ("index (row)") 7 ("index (row)") 7 ("index (row)") 7 ("index (row)") 7 ("index (row)")] -> w776
          tunnel: [-1000 ("disabled index (col)") 0 ("disabled index (col)") 1 ("disabled index (col)") 2 ("disabled index (col)") 3 ("disabled index (col)") 4 ("disabled index (col)") 5 ("disabled index (col)") 6 ("disabled index (col)") 7 ("disabled index (col)") 0 ("disabled index (col)") 1 ("disabled index (col)") 2 ("disabled index (col)") 3 ("disabled index (col)") 4 ("disabled index (col)") 5 ("disabled index (col)") 6 ("disabled index (col)") 7 ("disabled index (col)") 0 ("disabled index (col)") 1 ("disabled index (col)") 2 ("disabled index (col)") 3 ("disabled index (col)") 4 ("disabled index (col)") 5 ("disabled index (col)") 6 ("disabled index (col)") 7 ("disabled index (col)") 0 ("disabled index (col)") 1 ("disabled index (col)") 2 ("disabled index (col)") 3 ("disabled index (col)") 4 ("disabled index (col)") 5 ("disabled index (col)") 6 ("disabled index (col)") 7 ("disabled index (col)") 0 ("disabled index (col)") 1 ("disabled index (col)") 2 ("disabled index (col)") 3 ("disabled index (col)") 4 ("disabled index (col)") 5 ("disabled index (col)") 6 ("disabled index (col)") 7 ("disabled index (col)") 0 ("disabled index (col)") 1 ("disabled index (col)") 2 ("disabled index (col)") 3 ("disabled index (col)") 4 ("disabled index (col)") 5 ("disabled index (col)") 6 ("disabled index (col)") 7 ("disabled index (col)") 0 ("disabled index (col)") 1 ("disabled index (col)") 2 ("disabled index (col)") 3 ("disabled index (col)") 4 ("disabled index (col)") 5 ("disabled index (col)") 6 ("disabled index (col)") 7 ("disabled index (col)") 0 ("disabled index (col)") 1 ("disabled index (col)") 2 ("disabled index (col)") 3 ("disabled index (col)") 4 ("disabled index (col)") 5 ("disabled index (col)") 6 ("disabled index (col)") 7 ("disabled index (col)")] -> w775
          event Timeout {
            n743 = event-data() -> ()  [unwired: 1 in, 3 out]
          }
          event "0 0": Mouse Down {
            n744 = event-data() -> ()  [unwired: 1 in, 8 out]
          }
          event "0 1": Mouse Down {
            n745 = event-data() -> ()  [unwired: 1 in, 8 out]
          }
          event "0 2": Mouse Down {
            n746 = event-data() -> ()  [unwired: 1 in, 8 out]
          }
          event "0 3": Mouse Down {
            n747 = event-data() -> ()  [unwired: 1 in, 8 out]
          }
          event "0 4": Mouse Down {
            n748 = event-data() -> ()  [unwired: 1 in, 8 out]
          }
          event "0 5": Mouse Down {
            n749 = event-data() -> ()  [unwired: 1 in, 8 out]
          }
          event "0 6": Mouse Down {
            n750 = event-data() -> ()  [unwired: 1 in, 8 out]
          }
          event "0 7": Mouse Down {
            n751 = event-data() -> ()  [unwired: 1 in, 8 out]
          }
          event "1 0": Mouse Down {
            n752 = event-data() -> ()  [unwired: 1 in, 8 out]
          }
          event "1 1": Mouse Down {
            n753 = event-data() -> ()  [unwired: 1 in, 8 out]
          }
          event "1 2": Mouse Down {
            n754 = event-data() -> ()  [unwired: 1 in, 8 out]
          }
          event "1 3": Mouse Down {
            n755 = event-data() -> ()  [unwired: 1 in, 8 out]
          }
          event "1 4": Mouse Down {
            n756 = event-data() -> ()  [unwired: 1 in, 8 out]
          }
          event "1 5": Mouse Down {
            n757 = event-data() -> ()  [unwired: 1 in, 8 out]
          }
          event "1 6": Mouse Down {
            n758 = event-data() -> ()  [unwired: 1 in, 8 out]
          }
          event "1 7": Mouse Down {
            n759 = event-data() -> ()  [unwired: 1 in, 8 out]
          }
          event "2 0": Mouse Down {
            n760 = event-data() -> ()  [unwired: 1 in, 8 out]
          }
          event "2 1": Mouse Down {
            n761 = event-data() -> ()  [unwired: 1 in, 8 out]
          }
          event "2 2": Mouse Down {
            n762 = event-data() -> ()  [unwired: 1 in, 8 out]
          }
          event "2 3": Mouse Down {
            n763 = event-data() -> ()  [unwired: 1 in, 8 out]
          }
          event "2 4": Mouse Down {
            n764 = event-data() -> ()  [unwired: 1 in, 8 out]
          }
          event "2 5": Mouse Down {
            n765 = event-data() -> ()  [unwired: 1 in, 8 out]
          }
          event "2 6": Mouse Down {
            n766 = event-data() -> ()  [unwired: 1 in, 8 out]
          }
          event "2 7": Mouse Down {
            n767 = event-data() -> ()  [unwired: 1 in, 8 out]
          }
          event "3 0": Mouse Down {
            n768 = event-data() -> ()  [unwired: 1 in, 8 out]
          }
          event "3 1": Mouse Down {
            n769 = event-data() -> ()  [unwired: 1 in, 8 out]
          }
          event "3 2": Mouse Down {
            n770 = event-data() -> ()  [unwired: 1 in, 8 out]
          }
          event "3 3": Mouse Down {
            n771 = event-data() -> ()  [unwired: 1 in, 8 out]
          }
          event "3 4": Mouse Down {
            n772 = event-data() -> ()  [unwired: 1 in, 8 out]
          }
          event "3 5": Mouse Down {
            n773 = event-data() -> ()  [unwired: 1 in, 8 out]
          }
          event "3 6": Mouse Down {
            n774 = event-data() -> ()  [unwired: 1 in, 8 out]
          }
          event "3 7": Mouse Down {
            n775 = event-data() -> ()  [unwired: 1 in, 8 out]
          }
          event "4 0": Mouse Down {
            n776 = event-data() -> ()  [unwired: 1 in, 8 out]
          }
          event "4 1": Mouse Down {
            n777 = event-data() -> ()  [unwired: 1 in, 8 out]
          }
          event "4 2": Mouse Down {
            n778 = event-data() -> ()  [unwired: 1 in, 8 out]
          }
          event "4 3": Mouse Down {
            n779 = event-data() -> ()  [unwired: 1 in, 8 out]
          }
          event "4 4": Mouse Down {
            n780 = event-data() -> ()  [unwired: 1 in, 8 out]
          }
          event "4 5": Mouse Down {
            n781 = event-data() -> ()  [unwired: 1 in, 8 out]
          }
          event "4 6": Mouse Down {
            n782 = event-data() -> ()  [unwired: 1 in, 8 out]
          }
          event "4 7": Mouse Down {
            n783 = event-data() -> ()  [unwired: 1 in, 8 out]
          }
          event "5 0": Mouse Down {
            n784 = event-data() -> ()  [unwired: 1 in, 8 out]
          }
          event "5 1": Mouse Down {
            n785 = event-data() -> ()  [unwired: 1 in, 8 out]
          }
          event "5 2": Mouse Down {
            n786 = event-data() -> ()  [unwired: 1 in, 8 out]
          }
          event "5 3": Mouse Down {
            n787 = event-data() -> ()  [unwired: 1 in, 8 out]
          }
          event "5 4": Mouse Down {
            n788 = event-data() -> ()  [unwired: 1 in, 8 out]
          }
          event "5 5": Mouse Down {
            n789 = event-data() -> ()  [unwired: 1 in, 8 out]
          }
          event "5 6": Mouse Down {
            n790 = event-data() -> ()  [unwired: 1 in, 8 out]
          }
          event "5 7": Mouse Down {
            n791 = event-data() -> ()  [unwired: 1 in, 8 out]
          }
          event "6 0": Mouse Down {
            n792 = event-data() -> ()  [unwired: 1 in, 8 out]
          }
          event "6 1": Mouse Down {
            n793 = event-data() -> ()  [unwired: 1 in, 8 out]
          }
          event "6 2": Mouse Down {
            n794 = event-data() -> ()  [unwired: 1 in, 8 out]
          }
          event "6 3": Mouse Down {
            n795 = event-data() -> ()  [unwired: 1 in, 8 out]
          }
          event "6 4": Mouse Down {
            n796 = event-data() -> ()  [unwired: 1 in, 8 out]
          }
          event "6 5": Mouse Down {
            n797 = event-data() -> ()  [unwired: 1 in, 8 out]
          }
          event "6 6": Mouse Down {
            n798 = event-data() -> ()  [unwired: 1 in, 8 out]
          }
          event "6 7": Mouse Down {
            n799 = event-data() -> ()  [unwired: 1 in, 8 out]
          }
          event "7 0": Mouse Down {
            n800 = event-data() -> ()  [unwired: 1 in, 8 out]
          }
          event "7 1": Mouse Down {
            n801 = event-data() -> ()  [unwired: 1 in, 8 out]
          }
          event "7 2": Mouse Down {
            n802 = event-data() -> ()  [unwired: 1 in, 8 out]
          }
          event "7 3": Mouse Down {
            n803 = event-data() -> ()  [unwired: 1 in, 8 out]
          }
          event "7 4": Mouse Down {
            n804 = event-data() -> ()  [unwired: 1 in, 8 out]
          }
          event "7 5": Mouse Down {
            n805 = event-data() -> ()  [unwired: 1 in, 8 out]
          }
          event "7 6": Mouse Down {
            n806 = event-data() -> ()  [unwired: 1 in, 8 out]
          }
          event "7 7": Mouse Down {
            n807 = event-data() -> ()  [unwired: 1 in, 8 out]
          }
        }
        n808 = local write "pressedJ"(w775) -> ()
        n809 = local write "pressedI"(w776) -> ()
        n810 = for {
          N: 8 -> [_]
          shift-right: [w787] -> w778
          shift-left: w779 -> [w788]
          tunnel: w777 -> [w784]
          i -> [w785]
          # "若有，則1:黑 0:白"
          # "有無棋子"
          n811 = local read "currentState.pos"() -> (w783:i32[][])
          n812 = local read "currentState.exist"() -> (w786:i32[][])
          n813 = for {
            N: 8 -> [_]
            shift-right: [w798] -> w787
            shift-left: w788 -> [w799]
            tunnel: w786 -> [w800]
            tunnel: w785 -> [w790]
            tunnel: w784 -> [w794]
            tunnel: w783 -> [w793]
            i -> [w791]
            n814 = Index Array(array=w800, index (row)=w790, index (col)=w791) -> (element=w795:i32)
            n815 = Index Array(array=w793, index (row)=w790, index (col)=w791) -> (element=w792:i32)
            n816 = Not Equal?(x=w795, y=0) -> (x != y?=w796:bool)
            n817 = case shown="True" w796 {
              tunnel: w791 -> [_ w809]
              tunnel: w790 -> [_ w808]
              tunnel: w799 -> [w801 w807]
              tunnel: [w801 w806] -> w798
              tunnel: w792 -> [_ w805]
              tunnel: w794 -> [_ w803]
              frame False {
              }
              frame True {
                # "在指定位置畫黑/白子"
                n818 = Greater?(x=w805, y=0.0) -> (0:w802:bool)
                n819 = call "putPiece(picture).vi"("drawRed"=w802, "posy"=w808, "posx"=w809, "picture size"=w803, "2D Picture 2"=w807) -> ("2D Picture"=w806:picture)  [unwired: 6 in]
              }
            }
          }
        }
        "board" <- w778
        n820 = Greater Than 0?(x=w773) -> (x > 0?=→"x > 0?":bool)
        n821 = local read "PowerOff"() -> (w774:bool)
        n822 = Wait Until Next ms Multiple(millisecond multiple=u32 200) -> ()  [unwired: 1 out]
      }
    }
  }
